vi "TLB Native Dynamic Events ver 0.14.vi"() -> ()   [LabVIEW 2018]
uses:
  Labview Training Phase 2/Enum Controls/States for Action Engine.ctl
  TLB Type Definitions/State Type Definitions.ctl
  TLB Type Definitions/Intruction Type Definitions.ctl
  TLB Type Definitions/Encoder cluster.ctl
  TLB Type Definitions/PING CLUSTER.ctl
  <vilib>/Studica/Studica Toolkit/NavX/NavX.lvlib
  <vilib>/Studica/Studica Toolkit/Background/DIO Channel.ctl
  Underlying VI's/NavX VI/navX type def.ctl
  <vilib>/myRIO/Instrument Drivers/Utilities/Utilities.lvlib
  <vilib>/Studica/Studica Toolkit/Background/I2C Channel.ctl
  TLB Type Definitions/Vision cluster.ctl
  <vilib>/NI_Real-Time Target Support.lvlib
  TLB Type Definitions/Stepper cluster.ctl
  Experimental VI's/Archived VI's/MOTOR CONTROL NO PID Type Def.ctl
  Underlying VI's/I2C Master VI/I2C MASTER Type Def.ctl
  Underlying VI's/I2C Master VI/I2C_MASTER_WRITE_NEW Type Def.ctl
  <vilib>/userdefined/High Color/IMAQdx.ctl
  Underlying VI's/I2C Master VI/Arduino_Interfacing.ctl
  TLB Type Definitions/Yaw Cluster.ctl
  Experimental VI's/Archived VI's/MOTOR CONTROL NO PID AE DATA ENTRY MODE Type def.ctl
  Experimental VI's/Archived VI's/MOTOR CONTROL NO PID AE DIRECTIONS type def.ctl
  Underlying VI's/Elasped Timer/Control.ctl
  TLB Type Definitions/Time cluster.ctl
  TLB Type Definitions/Y Stepper cluster.ctl
  Underlying VI's/Modified webcam FGV/Webcam AE.ctl
  <vilib>/Utility/RT CPU Load.ctl
panel:
  out "Object Center Coordinates":cluster{"x":sgl, "y":sgl}
  out "Object detection cluster":T1
  out "Time up flag":bool
  out "Speed & distance":T2
  out "Task selection":u8
  in  "Object recognition mode":enum16{"Ball", "Soap", "Gel", "Pipe", "None"}(ring)
  out "NavX Readings":T3
  out "Arduino Data":T4
  out "CPU loads":T5[](array[typedef]) {"ISR (%)" format="%#.2f"; "Idle (%)" format="%#.2f"; "Background (%)" format="%#.2f"; "Normal (%)" format="%#.2f"; "Above Normal (%)" format="%#.2f"; "High (%)" format="%#.2g"; "Timed Structures (%)" format="%#.2g"; "Time Critical (%)" format="%#.2g"; "Total (%)" format="%#.2g"}
  in  "Red LED":bool
  out "Obstacle detected?":bool
  out "TASK ENABLE":bool
  out "Rising Edge":bool
  in  "Green LED":bool
  out "Obstacle detected":bool
  out "I2C Error":errorcluster
  out "State Logic":T6=enum."Startup"
  out "elements":T7[](array[typedef])
  in  "STOP TASK":bool
  in  "OK Button":bool
  in  "STOP":bool
  out "error out":errorcluster
  out "Action Queue Items":i32
  out "State Logic Queue Items":i32
  out "Action Queues items":string[](array[string])=["Hardware reset", "Software reset", ""]
  out "Action State":string
  # "VISION"
  # "System Health Status Update"
  # "TLB FRAMEWORK STATUS"
  # "Test Programme written by Calvin Loke    Dated: 28 Aug 2019\nTest Programme revised by Dr Alex See   Dated 30 Aug 2019\n\nRevision date: 20/03/2020\nProgramme version:   TLB Native Dynamic Events ver 0.14"
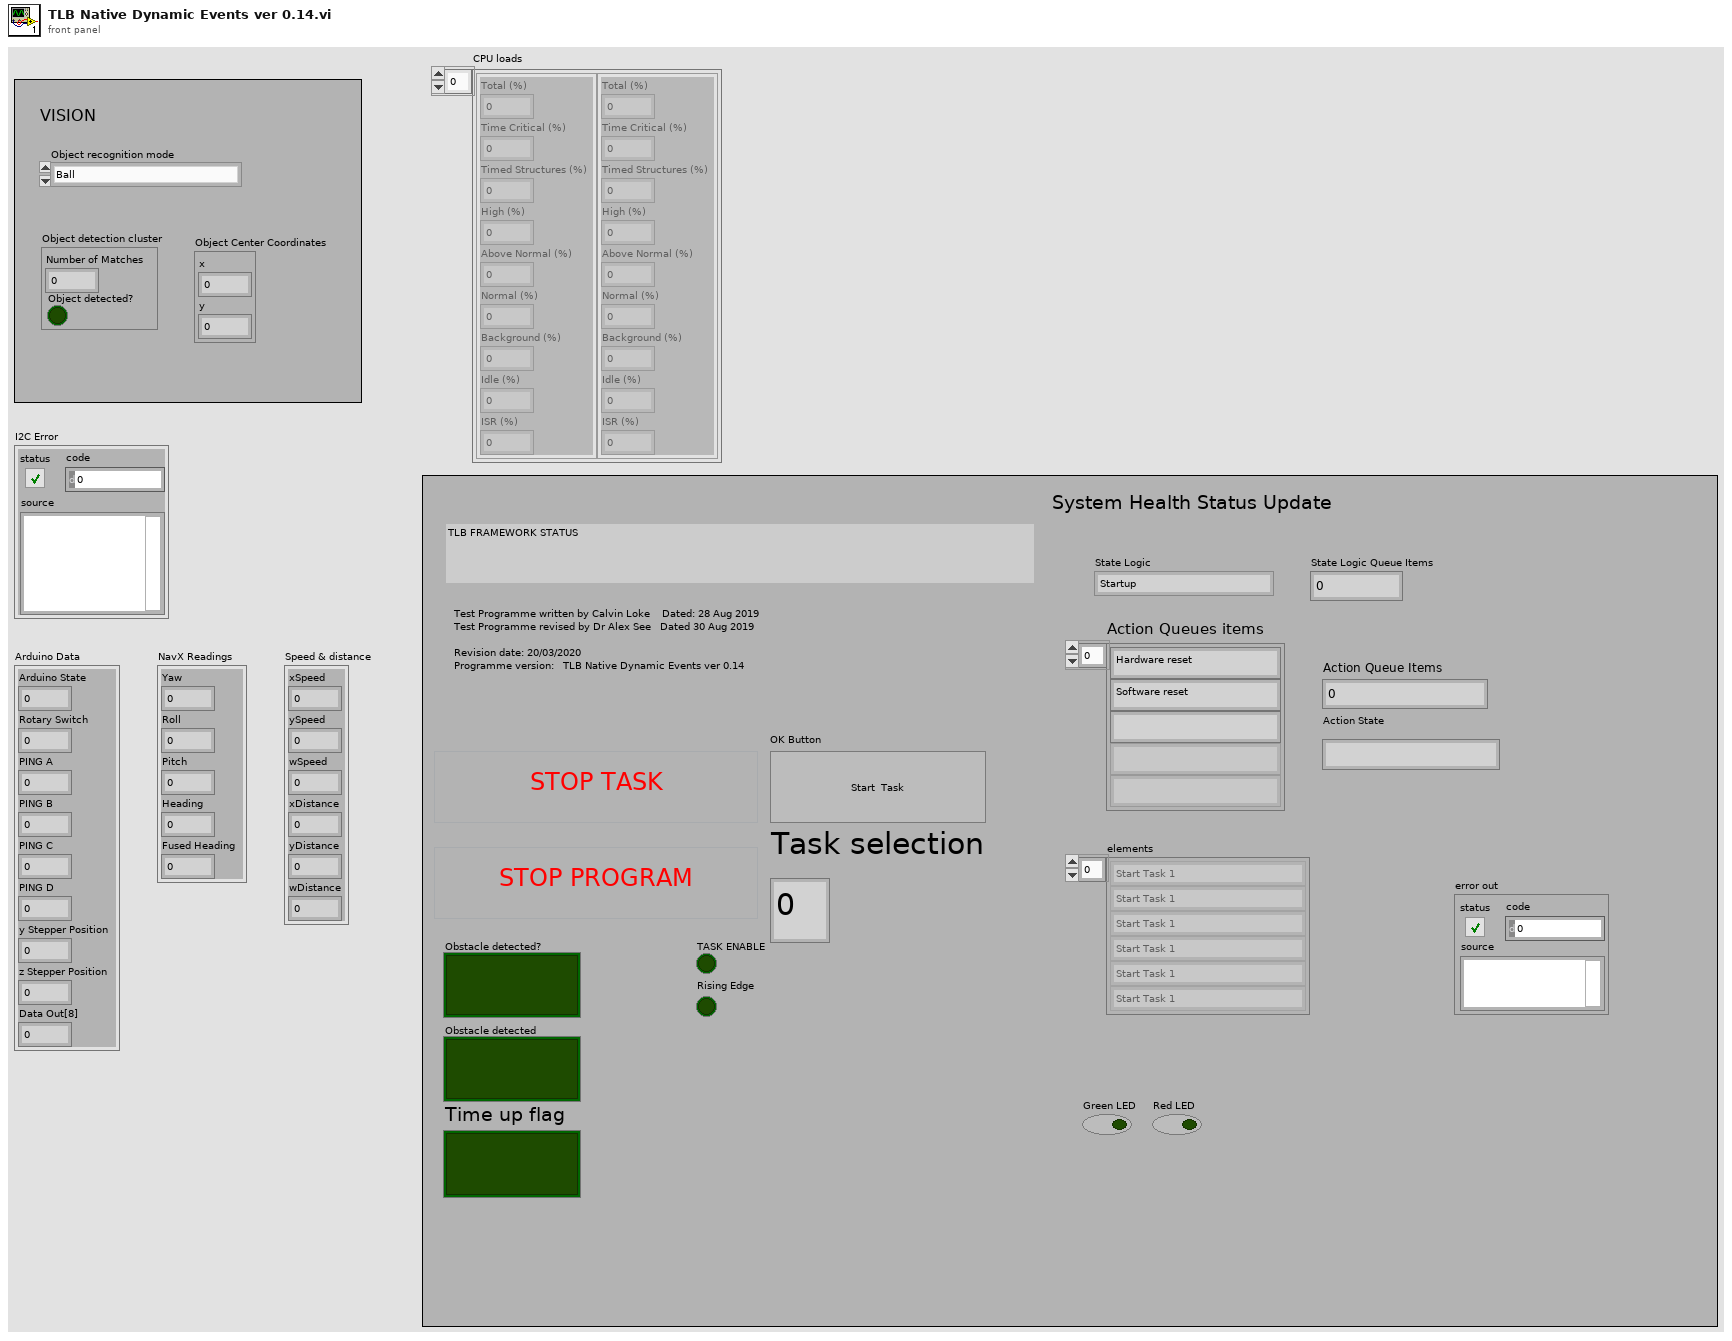
[diagram p1: front panel]
types:
  T1 = cluster{"Number of Matches":i32, "Object detected?":bool}
  T2 = cluster{"xSpeed":dbl, "ySpeed":dbl, "wSpeed":dbl, "xDistance":dbl, "yDistance":dbl, "wDistance":dbl}
  T3 = cluster{"Yaw":dbl, "Roll":dbl, "Pitch":dbl, "Heading":dbl, "Fused Heading":dbl}
  T4 = cluster{"Arduino State":u8, "Rotary Switch":u8, "PING A":u8, "PING B":u8, "PING C":u8, "PING D":u8, "y Stepper Position":u8, "z Stepper Position":u8, "Data Out[8]":u8}
  T5 = typedef "NI_Real-Time Target Support.lvlib/RT CPU Load.ctl" = cluster{"Total (%)":dbl, "Time Critical (%)":dbl, "Timed Structures (%)":dbl, "High (%)":dbl, "Above Normal (%)":dbl, "Normal (%)":dbl, "Background (%)":dbl, "Idle (%)":dbl, "ISR (%)":dbl}
  T6 = typedef "State Type Definitions.ctl" = enum16{"None", "Startup", "Move to Angle", "True Stop", "Idle", "Shutdown", "Task 1A", "Task 1B", "Task 2:Raise Arm", "Task 2:Sensor Mode", "Task 2:Reverse Mode", "Task 3", "Task 4_A", "Task 4_B", "Task 4_C", "Task 4_D", "Task 5A", "Task 5B", "Task 5C", "Task 5D", "Task 5E: POSITION ARM", "Task 5F: ARM GRAB HEIGHT", "Task 5G: CLOSE CLAW", "Task 5H: RAISE ARM", "Task 6_A", "Task 6_B", "Task 7", "Task 8A: RAISE ARM", "Task 8B: MOVE TO BOX", "Task 8C: CAM BURST", "Task 8D: PROCESS IMAGE", "Task 8E: ROBOT ADJUST", "Task 8F: CAM BURST 2", "Task 8G: PROCESS IMAGE 2", "Task 8H: ARM ADJUST", "Task 8I: ARM GRAB HEIGHT", "Task 8J: CLOSE CLAW", "Task 8K: RAISE MY SWORD", "Task 9A: Raise Arm", "Task 9B: Rotate to Angle", "Task 9C: Detect Box", "Task 9D: MOVE FORWARD", "Task 9E: MOVE LEFT", "Task 9F: SCAN IMAGE", "Task 9G: PROCESS COLOUR", "Task 9H: MOVE RIGHT", "Task 9I: SCAN IMAGE", "Task 9J: PROCESS COLOUR", "Task 9K: ROTATE 90 CW", "Task 9L: MOVE FORWARD", "Task 9M: MOVE RIGHT", "Task 9N: SCAN IMAGE", "Task 9O: PROCESS COLOUR", "Task 9P: MOVE RIGHT", "Task 9Q: SCAN IMAGE", "Task 9R: PROCESS COLOUR", "Task A1: Raise Arm", "Task A2: Rotate to Angle", "Task A3: Move Forward", "Task A4: Rotate CW 90"}
  T7 = typedef "Intruction Type Definitions.ctl" = enum16{"None", "Start Task 1", "Start Task 2", "Start Task 3", "Start Task 4", "Start Task 5", "Start Task 6", "Start Task 7", "Start Task 8 - BALL", "Start Task 8 - Gel", "Start Task 8 - Pipe", "Start Task 8 - Soap", "Start Task 9", "Start Task A", "Start Task B", "Exit"}
  T8 = typedef "Y Stepper cluster.ctl" = cluster{"yStepper desired":u8}
  T9 = typedef "Time cluster.ctl" = cluster{"Time up flag":bool, "SET TIME TO CHECK":dbl}
  T10 = typedef "Yaw Cluster.ctl" = cluster{"Yaw":dbl, "Compass":dbl}
  T11 = typedef "Stepper cluster.ctl" = cluster{"y Stepper Position":u8, "z Stepper Position":u8}
  T12 = typedef "DIO Channel.ctl" = enum16{"Not Connected", "A/DIO1", "A/DIO2", "A/DIO3", "A/DIO4", "A/DIO5", "A/DIO6", "A/DIO7", "A/DIO13", "B/DIO1", "B/DIO2", "B/DIO3", "B/DIO4", "B/DIO5", "B/DIO6", "B/DIO7", "B/DIO13", "C/DIO0", "C/DIO1", "C/DIO2", "C/DIO3", "C/DIO4", "C/DIO5", "C/DIO6", "C/DIO7"}
  T13 = typedef "Vision cluster.ctl" = cluster{"Recognized Object":bool, "Object X coordinate":dbl, "Object Y coordinate":dbl}
  T14 = typedef "PING CLUSTER.ctl" = cluster{"PING_A":u8, "PING_B":u8, "PING_C":u8, "PING_D":u8}
  T15 = typedef "Encoder cluster.ctl" = cluster{"xDistance":dbl, "yDistance":dbl, "wDistance":dbl}
  T16 = cluster{"DIO Channel":T12, "FPGA VI Reference Out":refnum<k20>}
  T17 = typedef "MOTOR CONTROL NO PID AE DATA ENTRY MODE Type def.ctl" = enum16{"Initialize", "Reset Encoders", "Write to motors", "Read from Encoders"}
  T18 = typedef "navX type def.ctl" = enum16{"Get i2C reference", "Read Values", "Zero Yaw"}
  T19 = typedef "Arduino_Interfacing.ctl" = enum16{"Initialize", "Write to Arduino", "Read From Arduino"}
  T20 = typedef "I2C Channel.ctl" = enum16{"Not Connected", "A", "B"}
  T21 = typedef "States for Action Engine.ctl" = enum16{"Initialize", "Write", "Read"}
  T22 = cluster{"I2C Ref Out":cluster{"I2C Channel":T20, "FPGA VI Reference Out":refnum<k20>}, "Connected":bool, "Slave Address (7-bit)":u8, "Registry":u8[]}
  T23 = typedef "IMAQ Image.ctl" = refnum<image>
  T24 = typedef "State Type Definitions.ctl" = enum16{"None", "Startup", "Move to Angle", "True Stop", "Idle", "Shutdown", "Task 1", "Task 2", "Task 3", "Task 4_A", "Task 4_B", "Task 4_C", "Task 4_D", "Task 5_A", "Task 5 _B", "Task 5_C", "Task 5_D", "Task 5_D_Error", "Task 5D_Error_Right", "Task 5D_Error_Left", "Task 5_E", "Task 5_F", "Task 5F_Error", "Task 5G", "Task 5H", "Task 6_A", "Task 6_B", "Task 7", "Task 8", "Task 9", "Task A", "Task B"}
  T25 = typedef "State Type Definitions.ctl" = enum16{"None", "Startup", "Move to Angle", "True Stop", "Idle", "Shutdown", "Task 1", "Task 2", "Task 3", "Task 4_A", "Task 4_B", "Task 4_C", "Task 5_A", "Task 5 _B", "Task 5_C", "Task 5_C_Error", "Task 6_A", "Task 6_B", "Task 7", "Task 8", "Task 9", "Task A", "Task B"}
  T26 = typedef "MOTOR CONTROL NO PID AE DIRECTIONS type def.ctl" = enum16{"y-axis movement", "x-axis movement", "Rotate", "Stop"}
  T27 = typedef "Control.ctl" = enum16{"Start", "Pause", "Initialize"}
  T28 = typedef "I2C_MASTER_WRITE_NEW Type Def.ctl" = enum16{"Ultrasonic sensors", "Stepper origin", "zStepper 13.3k", "zStepper 13k", "zStepper 12k", "zStepper 11k", "zStepper 10k", "zStepper 9k", "zStepper 8k", "zStepper 7k", "zStepper 6k", "zStepper 5k", "zStepper 4k", "zStepper 3k", "zStepper 2k", "zStepper 1k", "zStepper 900", "zStepper 800", "zStepper 700", "zStepper 600", "zStepper 500", "zStepper 400", "zStepper 300", "zStepper 200", "zStepper 100", "zStepper 0", "yStepper control", "Open Claw", "Close Claw", "Soft Reset"}
  T29 = typedef "Webcam AE.ctl" = enum16{"Initialize Camera", "Open Camera", "Continuous Acquisition", "Close Camera", "Retrieve Image", "Dispose Camera Image Buffer"}
  T30 = typedef "IMAQdx.ctl" = refnum<k21>
  T31 = typedef "Webcam AE.ctl" = enum16{"Initialize Camera", "Open Camera", "Continuous Acquisition", "Close Camera", "Retrieve Image", "Dispose Image Buffers"}
  T32 = typedef "MOTOR CONTROL NO PID Type Def.ctl" = enum16{"Init", "Front Back", "Left Right", "Rotate", "Stop", "Latch"}
  T33 = typedef "I2C MASTER Type Def.ctl" = enum16{"Last State", "Mode 0", "Mode 1", "Mode 2", "Mode 3", "Mode 4", "Mode 5", "Mode 6", "Mode 7", "Mode 8", "Mode 9", "Mode 10"}
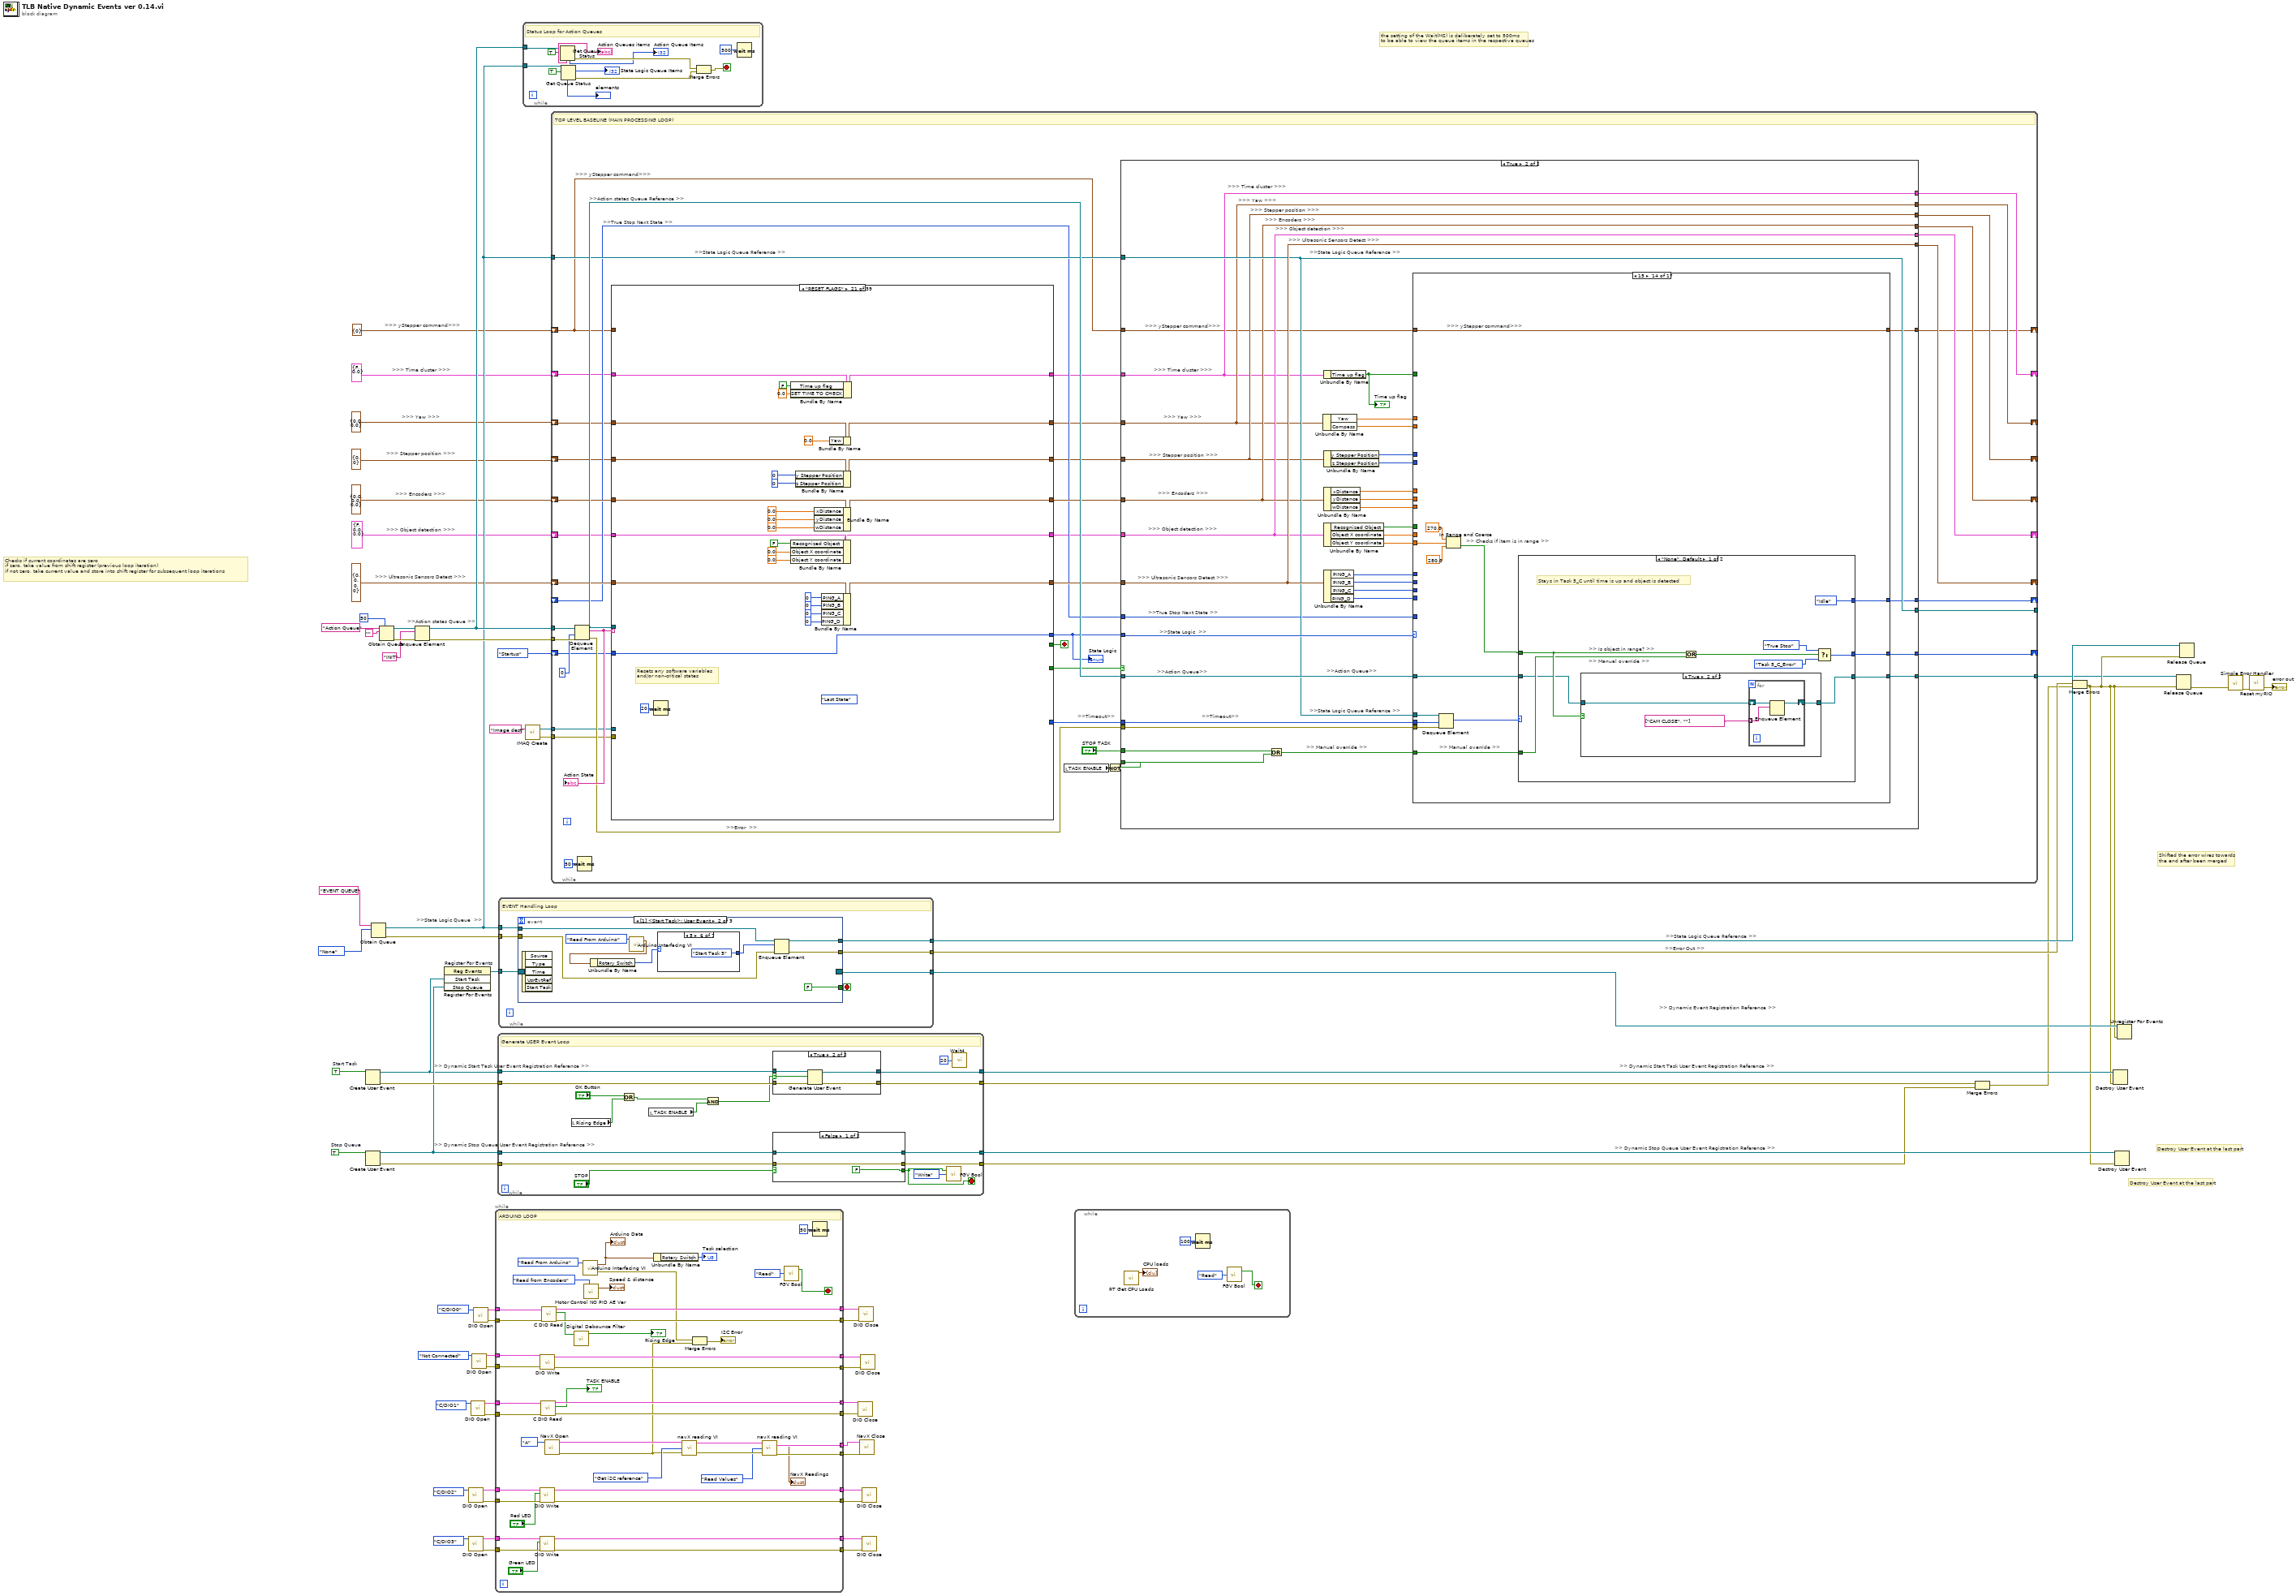
[diagram p0: block diagram]
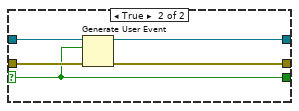
[diagram p2: hidden frame]
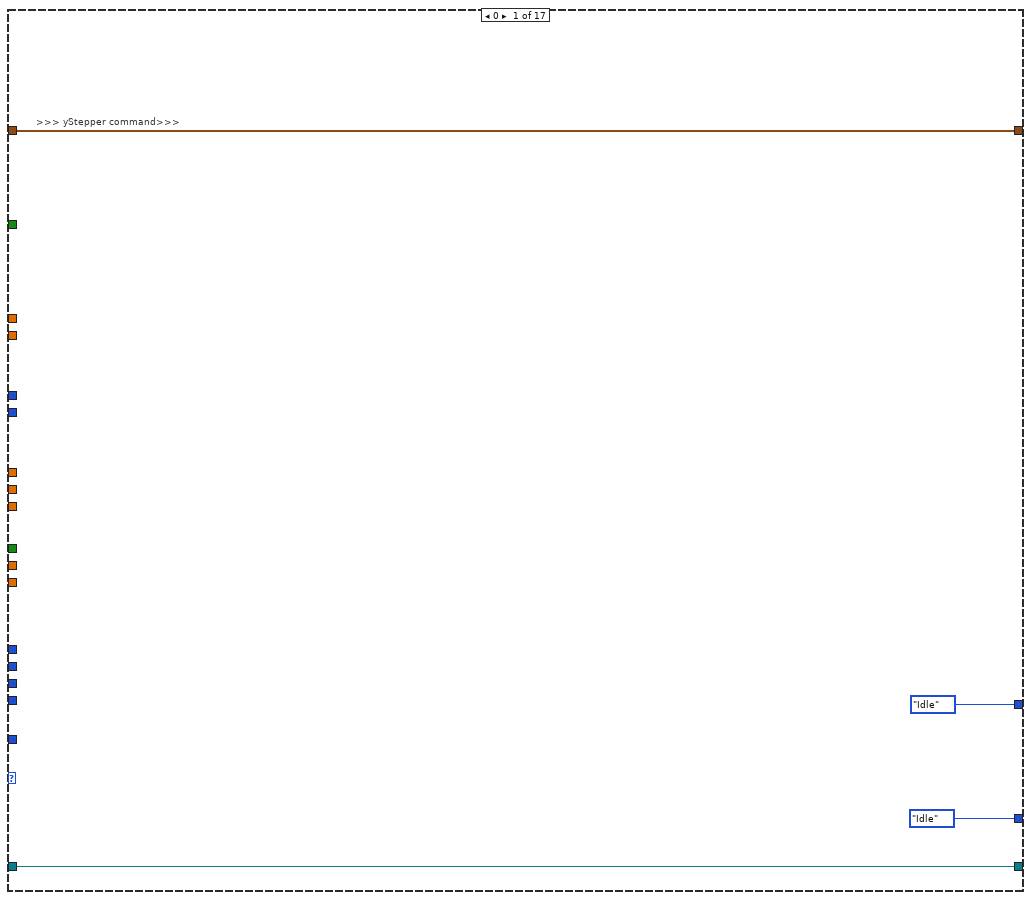
[diagram p5: hidden frame]
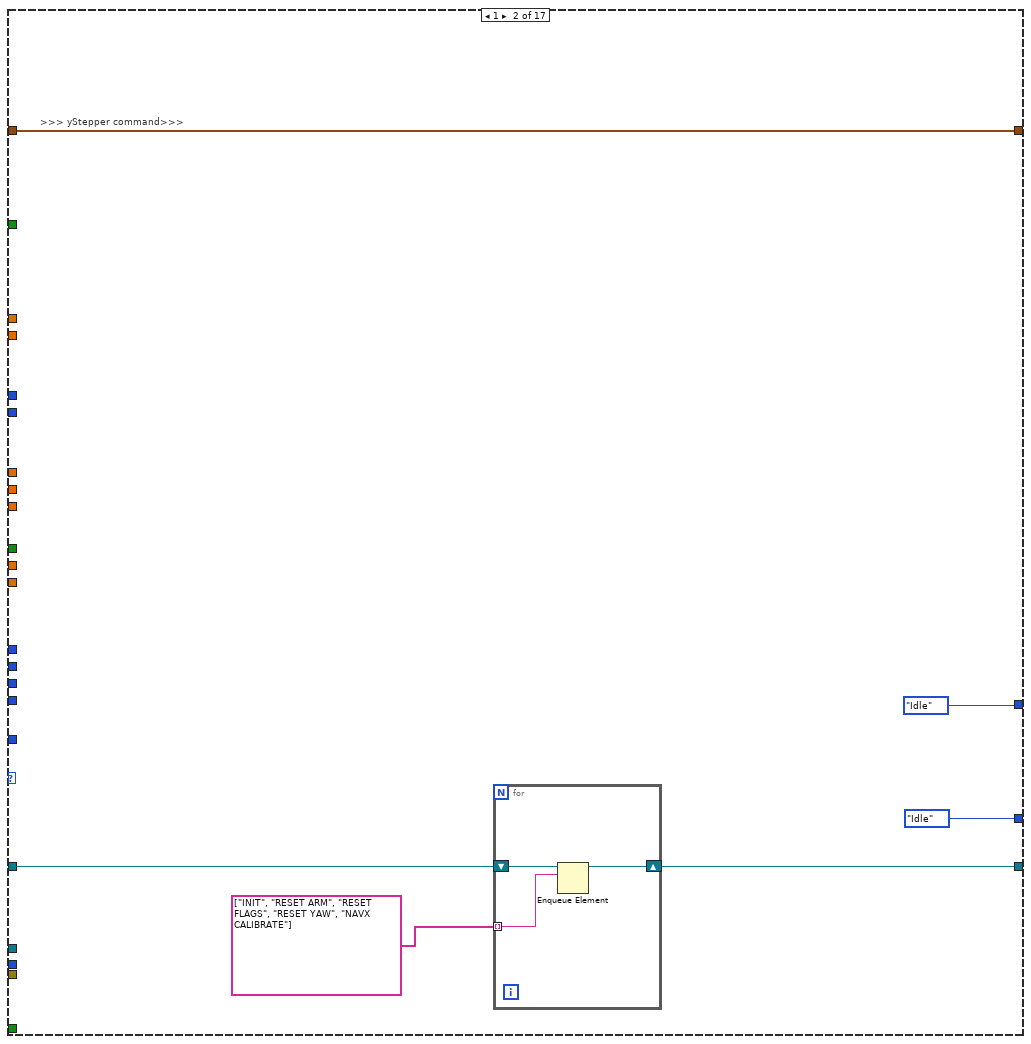
[diagram p6: hidden frame]
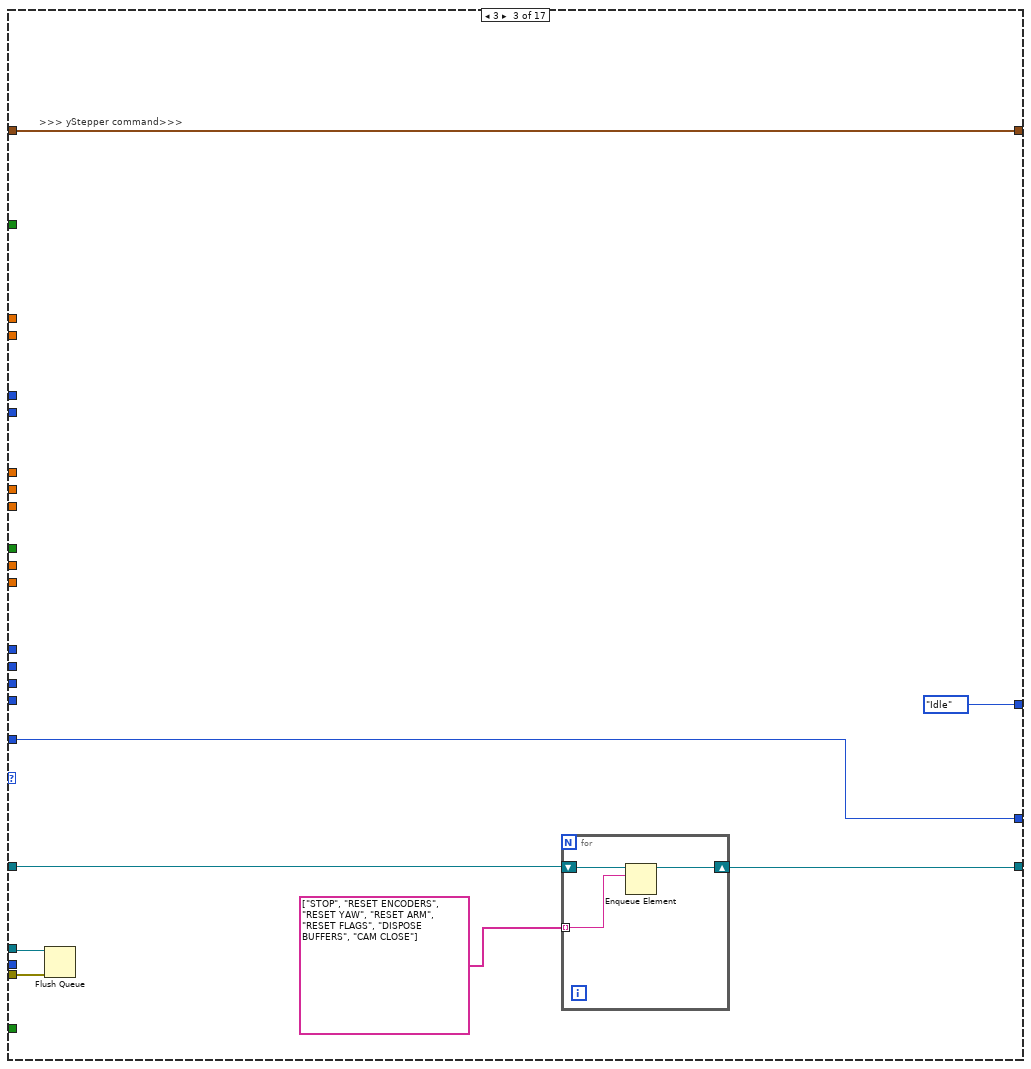
[diagram p7: hidden frame]
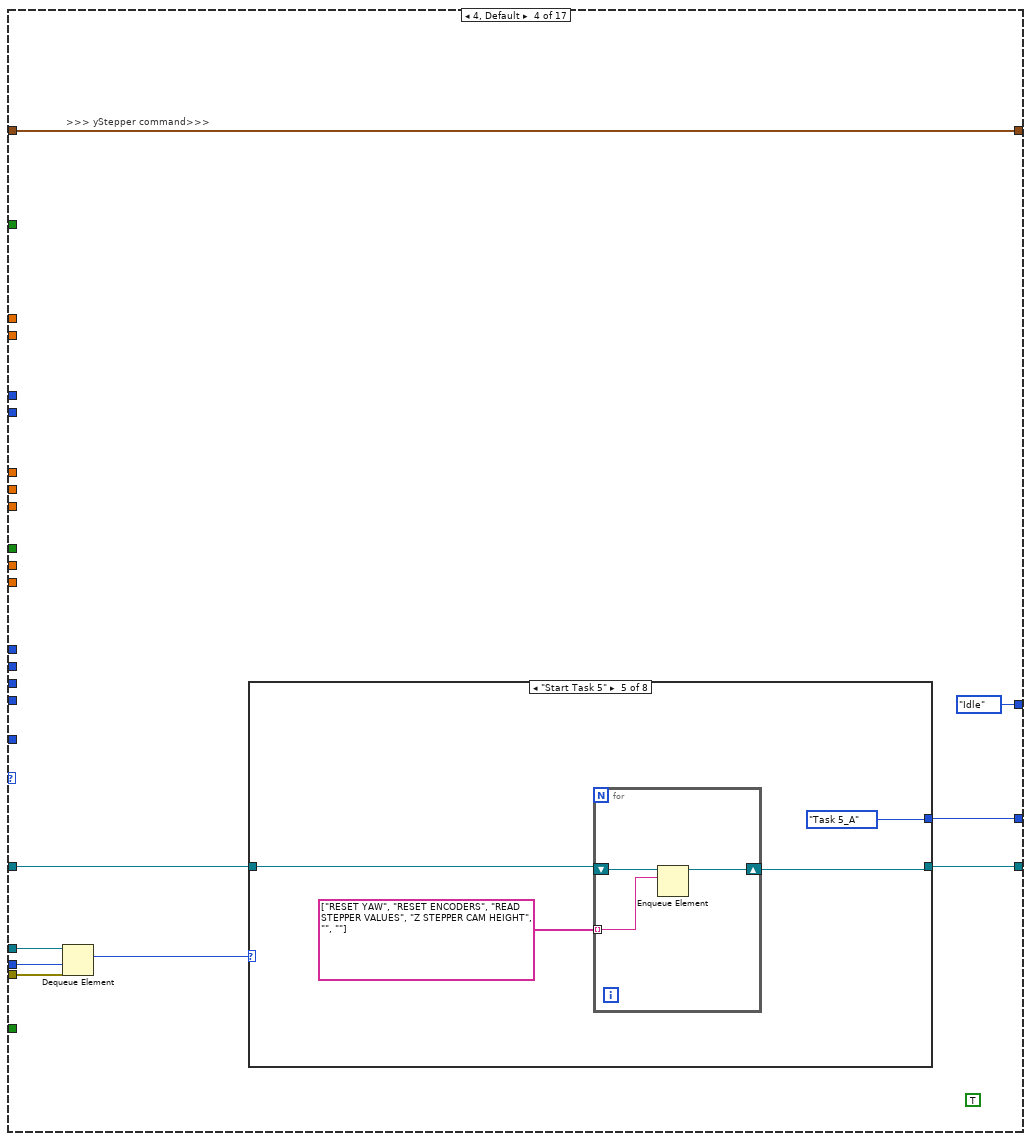
[diagram p8: hidden frame]
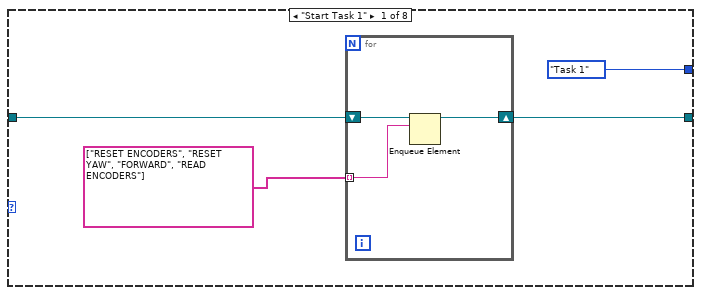
[diagram p9: hidden frame]
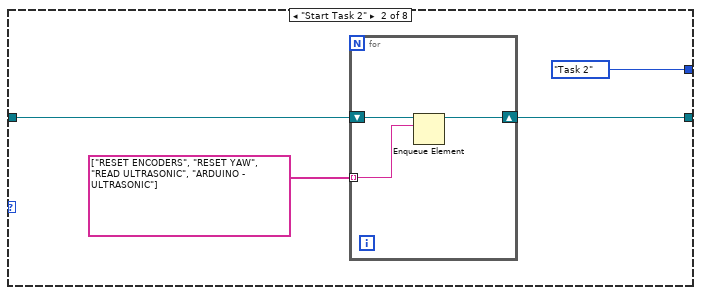
[diagram p10: hidden frame]
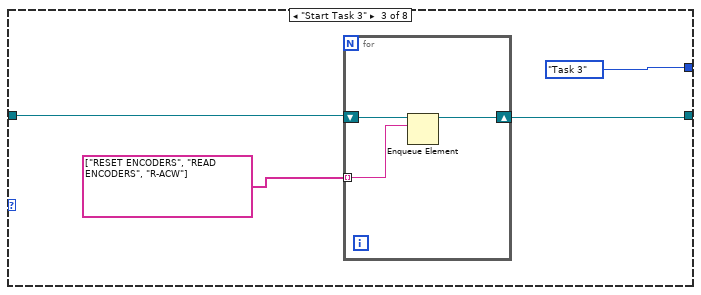
[diagram p11: hidden frame]
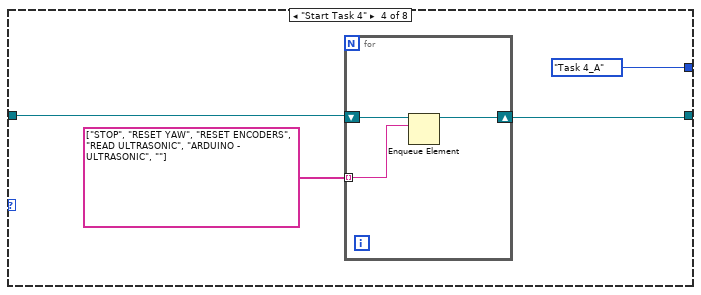
[diagram p12: hidden frame]
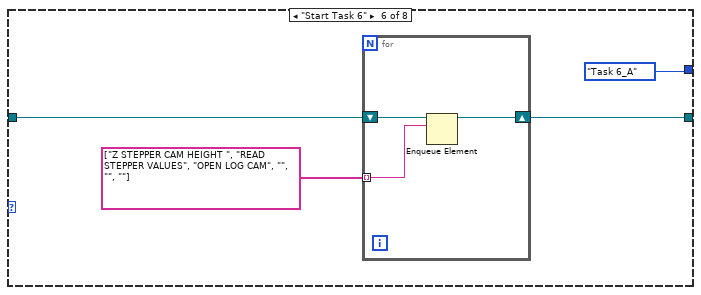
[diagram p13: hidden frame]
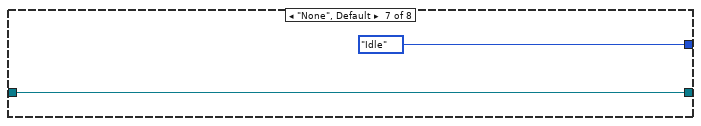
[diagram p14: hidden frame]
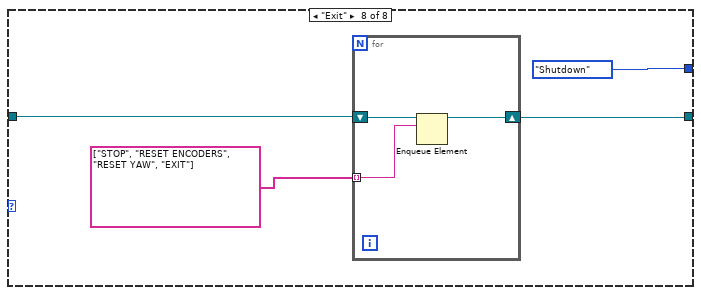
[diagram p15: hidden frame]
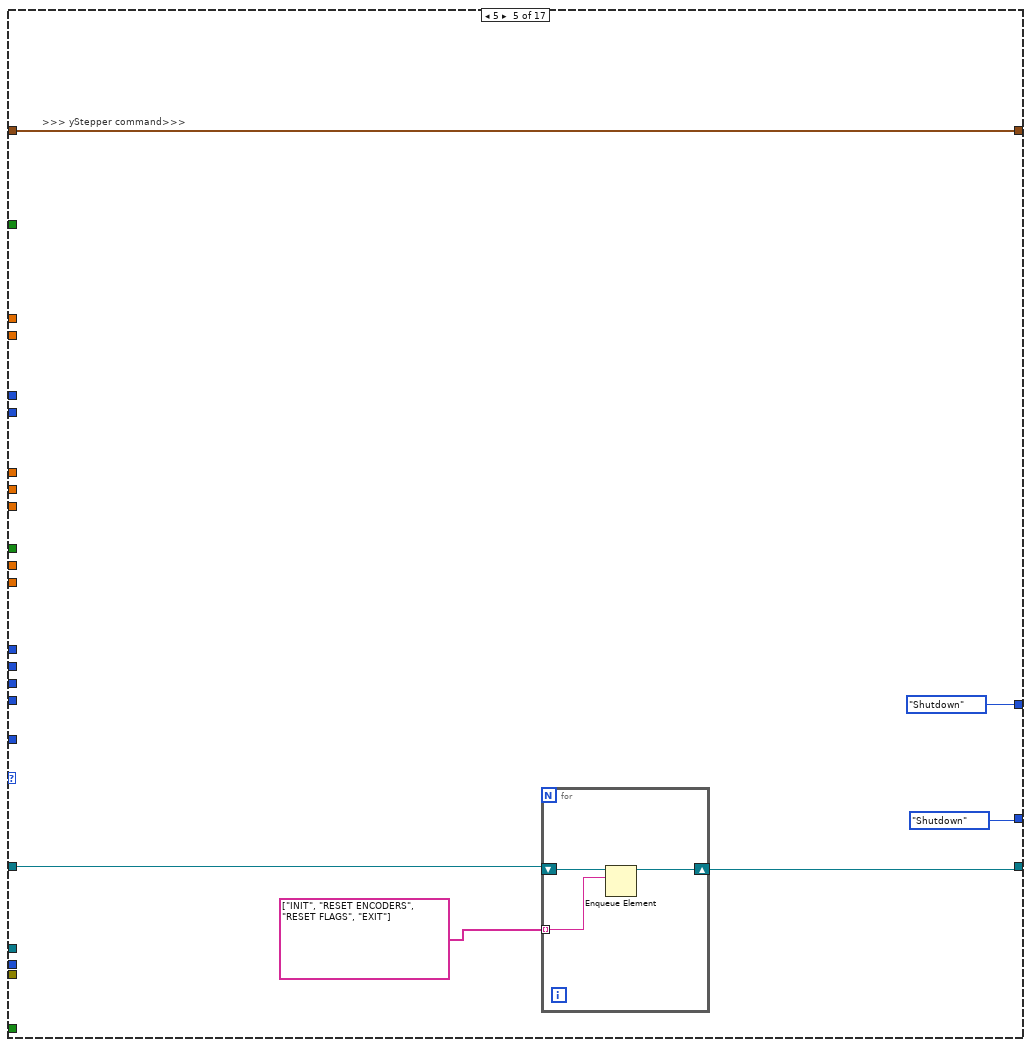
[diagram p16: hidden frame]
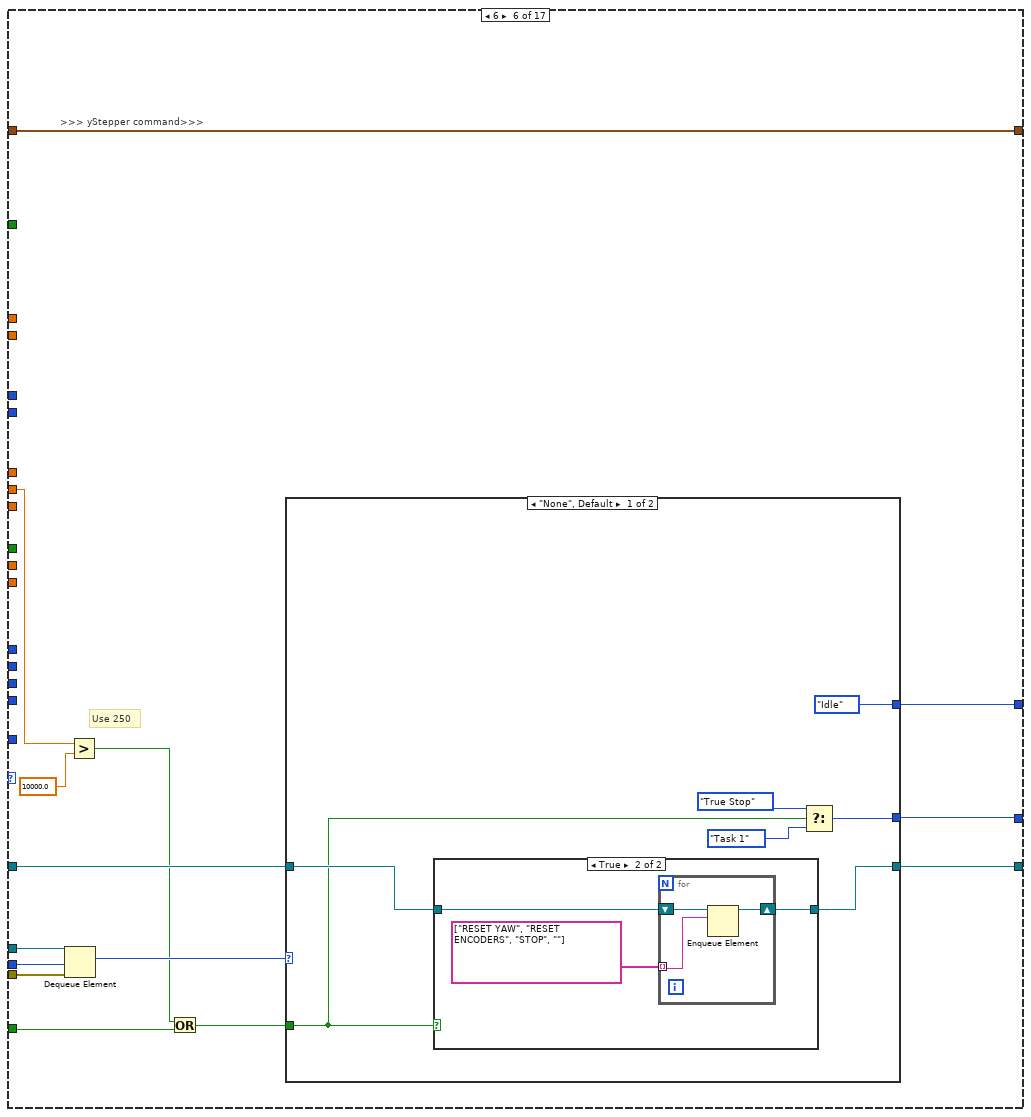
[diagram p17: hidden frame]
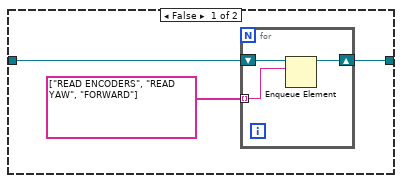
[diagram p18: hidden frame]
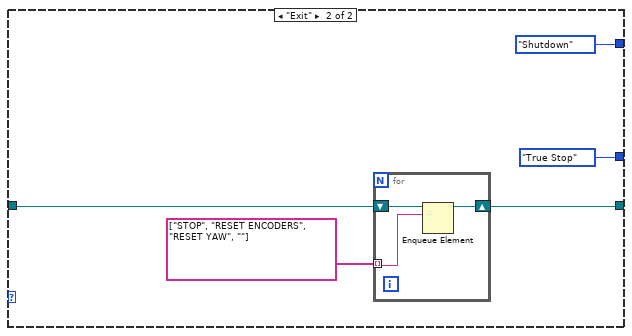
[diagram p19: hidden frame]
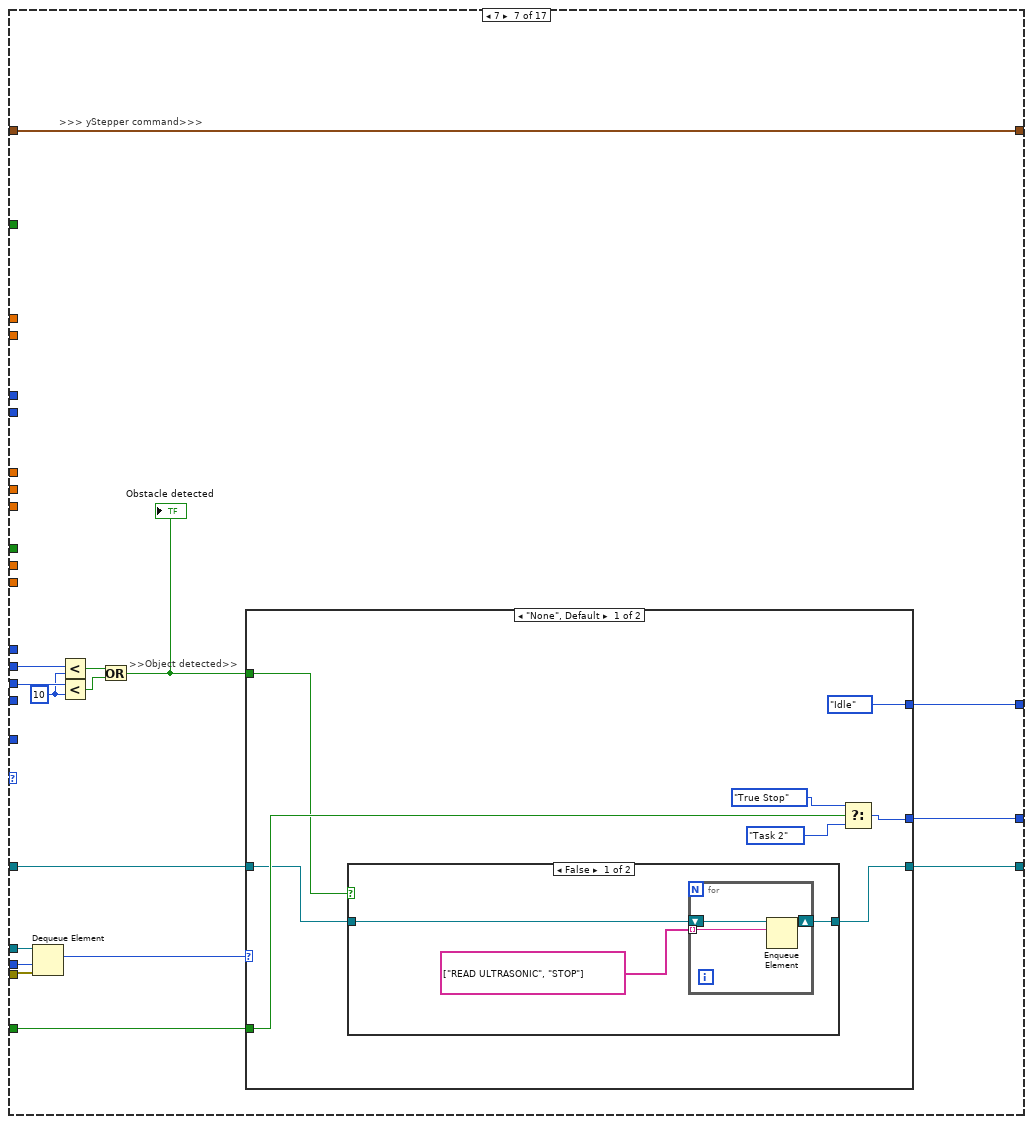
[diagram p20: hidden frame]
diagram:
  w70 = TRUE  # Stop Queue
  w69 = TRUE  # Start Task
  # "Checks if current coordinates are zero\nif zero, take value from shift register (previous loop iteration)\nif not zero, take current value and store into shift register for subsequent loop iterations"
  # ">>> yStepper command>>>"
  # ">>> Time cluster >>>"
  # ">>> Yaw >>>"
  # ">>> Stepper position >>>"
  # ">>> Encoders >>>"
  # ">>> Object detection >>>"
  # ">>> Ultrasonic Sensors Detect >>>"
  # "the setting of the Wait(MS) is deliberately set to 500ms\nto be able to view the queue items in the respective queues"
  # ">>Error Out >>"
  # ">> Dynamic Stop Queue User Event Registration Reference >>"
  # ">> Dynamic Start Task User Event Registration Reference >>"
  # ">> Dynamic Stop Queue User Event Registration Reference >>"
  # ">> Dynamic Start Task User Event Registration Reference >>"
  # ">> Dynamic Event Registration Reference >>"
  # ">>Action states Queue >>"
  # ">>State Logic Queue  >>"
  # ">>State Logic Queue Reference >>"
  # "Destroy User Event at the last part"
  # "Destroy User Event at the last part"
  # "Shifted the error wires towards\nthe end after been merged"
  n1 = Create User Event(user event datatype=w69) -> (user event=w61:refnum<user-event>, error out=w66:errorcluster)  [unwired: 1 in]
  n2 = Create User Event(user event datatype=w70) -> (user event=w62:refnum<user-event>, error out=w65:errorcluster)  [unwired: 1 in]
  n3 = Obtain Queue(name (unnamed)="EVENT QUEUE", element data type=Intruction_Type_Definitions."None" ("Enum")) -> (queue out=w47:refnum<queue>, error out=w53:errorcluster)  [unwired: 3 in, 1 out]
  n4 = Obtain Queue(max queue size (-1, unlimited)=50, name (unnamed)="Action Queue", element data type="") -> (queue out=w56:refnum<queue>, error out=w52:errorcluster)  [unwired: 2 in, 1 out]
  n5 = Enqueue Element(queue=w56, element="INIT", error in (no error)=w52) -> (queue out=w48:refnum<queue>, error out=w51:errorcluster)  [unwired: 1 in, 1 out]
  n6 = register-events "Register For Events"(w61, w62) -> (reference out=w60:refnum<event-registration>)  [unwired: 2 in, 1 out]
  n7 = call <vilib>:"DIO Open.vi"("DIO Channel"=DIO_Channel."C/DIO2") -> ("error out"=w14:errorcluster, "DIO Info Out"=w15:T16)  [unwired: 9 in]
  n8 = call <vilib>:"DIO Open.vi"("DIO Channel"=DIO_Channel."C/DIO3") -> ("error out"=w9:errorcluster, "DIO Info Out"=w10:T16)  [unwired: 9 in]
  n9 = call <vilib>:"DIO Open.vi"("DIO Channel"=DIO_Channel."C/DIO1") -> ("error out"=w25:errorcluster, "DIO Info Out"=w26:T16)  [unwired: 9 in]
  n10 = call <vilib>:"DIO Open.vi"("DIO Channel"=DIO_Channel."Not Connected") -> ("error out"=w30:errorcluster, "DIO Info Out"=w32:T16)  [unwired: 9 in]
  n11 = call <vilib>:"DIO Open.vi"("DIO Channel"=DIO_Channel."C/DIO0") -> ("error out"=w35:errorcluster, "DIO Info Out"=w38:T16)  [unwired: 9 in]
  n12 = while {
    tunnel: w38 -> [w112]
    tunnel: [w111] -> w36
    tunnel: w35 -> [w110]
    tunnel: [w109] -> w34
    tunnel: w32 -> [w105]
    tunnel: [w104] -> w31
    tunnel: w30 -> [w103]
    tunnel: [w102] -> w29
    tunnel: [w101] -> w27
    tunnel: w26 -> [w100]
    tunnel: w25 -> [w99]
    tunnel: [w98] -> w24
    tunnel: w15 -> [w92]
    tunnel: w14 -> [w91]
    tunnel: [w90] -> w13
    tunnel: [w89] -> w12
    tunnel: w10 -> [w87]
    tunnel: w9 -> [w86]
    tunnel: [w85] -> w8
    tunnel: [w84] -> w7
    tunnel: [w78] -> w4
    tunnel: [w77] -> w5
    stop <- w114 stop-if-true
    # "ARDUINO LOOP"
    n13 = call <vilib>:"DIO Write.vi"("error in (no error)"=w91, "Input"="Red LED", "DIO Info In"=w92) -> ("error out"=w89:errorcluster, "DIO Info Out"=w90:T16)  [unwired: 7 in]
    n14 = call <vilib>:"DIO Write.vi"("error in (no error)"=w86, "Input"="Green LED", "DIO Info In"=w87) -> ("error out"=w84:errorcluster, "DIO Info Out"=w85:T16)  [unwired: 7 in]
    n15 = call <vilib>:"DIO Write.vi"("error in (no error)"=w103, "DIO Info In"=w105) -> ("error out"=w102:errorcluster, "DIO Info Out"=w104:T16)  [unwired: 8 in]
    n16 = call <vilib>:"C DIO Read.vi"("error in (no error)"=w99, "DIO Info In in"=w100) -> ("error out"=w98:errorcluster, "IN"=→"TASK ENABLE":bool, "DIO Info In out"=w101:T16)  [unwired: 7 in]
    n17 = call <vilib>:"C DIO Read.vi"("error in (no error)"=w110, "DIO Info In in"=w112) -> ("error out"=w109:errorcluster, "IN"=w107:bool, "DIO Info In out"=w111:T16)  [unwired: 7 in]
    n18 = call <vilib>:"NavX Open.vi"("I2C Channel"=I2C_Channel."A") -> ("error out"=w94:errorcluster, "NavX Info"=w96:T22)  [unwired: 9 in]
    n19 = call "Digital Debounce Filter.vi"("Boolean input"=w107) -> ("Rising Edge"=→"Rising Edge":bool)  [unwired: 1 in, 2 out]
    n20 = call "Arduino Interfacing VI.vi"("AE Mode"=Arduino_Interfacing."Read From Arduino") -> ("error out"=w81:errorcluster, "Arduino Data"=w74:T4)  [unwired: 3 in]
    "Arduino Data" <- w74
    n21 = call "Motor Control NO PID AE Ver.vi"("AE Mode"=MOTOR_CONTROL_NO_PID_AE_DATA_ENTRY_MODE_Type_def."Read from Encoders") -> ("Speed & distance"=→"Speed & distance":T2)  [unwired: 4 in, 1 out]
    n22 = Unbundle By Name(w74) -> ("Rotary Switch"=→"Task selection":u8)
    n23 = call "navX reading VI.vi"("NavX Info In"=w96, "Mode"=navX_type_def."Get i2C reference", "error in (no error)"=w94) -> ("NavX Info Out"=w80:T22, "Error Out"=w79:errorcluster)  [unwired: 2 out]
    n24 = Merge Errors(w81, w94) -> (→"I2C Error":errorcluster)
    n25 = call "navX reading VI.vi"("NavX Info In"=w80, "Mode"=navX_type_def."Read Values", "error in (no error)"=w79) -> ("NavX Info Out"=w78:T22, "NavX Readings"=→"NavX Readings":T3, "Error Out"=w77:errorcluster)  [unwired: 1 out]
    n26 = call "FGV Bool.vi"("Init/Read/Write State"=States_for_Action_Engine."Read") -> ("Output node"=w114:bool)  [unwired: 2 in, 1 out]
    n27 = Wait (ms)(milliseconds to wait=u32 50) -> ()  [unwired: 1 out]
  }
  n28 = while {
    tunnel: w61 -> [w132]
    tunnel: w62 -> [w131]
    tunnel: [w130] -> w68
    tunnel: [w129] -> w67
    tunnel: w66 -> [w128]
    tunnel: [w127] -> w64
    tunnel: w65 -> [w126]
    tunnel: [w125] -> w63
    stop <- w123 stop-if-true
    # "Generate USER Event Loop"
    n29 = local read "Rising Edge"() -> (w119:bool)
    n30 = Or(x="OK Button", y=w119) -> (x .or. y?=w118:bool)
    n31 = local read "TASK ENABLE"() -> (w117:bool)
    n32 = And(x=w118, y=w117) -> (x .and. y?=w116:bool)
    n33 = case shown="True" w116 {
      selector: w116 -> [_ w143]
      tunnel: w132 -> [w142 w147]
      tunnel: [w142 w146] -> w129
      tunnel: w128 -> [w141 w145]
      tunnel: [w141 w144] -> w127
      frame False {
      }
      frame True {
        n34 = Generate User Event(user event=w147, event data cluster=w143, error in=w145) -> (user event out=w146:refnum<user-event>, error out=w144:errorcluster)  [unwired: 1 in]
      }
    }
    n35 = case shown="False" "STOP" {
      selector: "STOP" -> [_ w136]
      tunnel: w131 -> [w135 w140]
      tunnel: [w135 w139] -> w130
      tunnel: w126 -> [w134 w138]
      tunnel: [w134 w137] -> w125
      tunnel: [FALSE w136] -> w123
      frame False {
      }
      frame True {
        n36 = Generate User Event(user event=w140, event data cluster=w136, error in=w138) -> (user event out=w139:refnum<user-event>, error out=w137:errorcluster)  [unwired: 1 in]
      }
    }
    n37 = call "FGV Bool.vi"("Init/Read/Write State"=States_for_Action_Engine."Write", "Input Node"=w123) -> ()  [unwired: 1 in, 2 out]
    n38 = call "Wait4"("Count(uSec)"=u32 20) -> ()  [unwired: 1 out]
  }
  n39 = while {
    tunnel: w60 -> [w154]
    tunnel: [w153] -> w59
    tunnel: w47 -> [w151]
    tunnel: [w150] -> w58
    tunnel: w53 -> [w149]
    tunnel: [w148] -> w50
    stop <- w152 stop-if-true
    # "EVENT Handling Loop"
    n40 = event shown="[1] <Start Task>: User Event" {
      selector: w154 -> [_ _ _]
      dyn-events: [_ _ _] -> w153
      timeout: _ -> [_ _ _]
      tunnel: [FALSE FALSE w182] -> w152
      tunnel: w151 -> [w159 w168 w180]
      tunnel: [w158 w167 w181] -> w150
      tunnel: w149 -> [w157 w166 w179]
      tunnel: [w156 w165 w178] -> w148
      event Timeout {
        n41 = event-data() -> ()  [unwired: 1 in, 3 out]
        n42 = Enqueue Element(queue=w159, element=Intruction_Type_Definitions."None" ("Enum"), error in (no error)=w157) -> (queue out=w158:refnum<queue>, error out=w156:errorcluster)  [unwired: 1 in, 1 out]
      }
      event User Event {
        n43 = event-data() -> ()  [unwired: 1 in, 5 out]
        n44 = call "Arduino Interfacing VI.vi"("AE Mode"=Arduino_Interfacing."Read From Arduino") -> ("Arduino Data"=w162:T4)  [unwired: 3 in, 1 out]
        n45 = Unbundle By Name(w162) -> ("Rotary Switch"=w161:u8)
        n46 = case shown="5" w161 {
          tunnel: [Intruction_Type_Definitions."None" ("Enum") Intruction_Type_Definitions."Start Task 1" ("Enum") Intruction_Type_Definitions."Start Task 2" ("Enum") Intruction_Type_Definitions."Start Task 3" ("Enum") Intruction_Type_Definitions."Start Task 4" ("Enum") Intruction_Type_Definitions."Start Task 5" ("Enum") Intruction_Type_Definitions."Start Task 6" ("Enum")] -> w164
          frame 0, Default {
          }
          frame 1 {
          }
          frame 2 {
          }
          frame 3 {
          }
          frame 4 {
          }
          frame 5 {
          }
          frame 6 {
          }
        }
        n47 = Enqueue Element(queue=w168, element=w164, error in (no error)=w166) -> (queue out=w167:refnum<queue>, error out=w165:errorcluster)  [unwired: 1 in, 1 out]
      }
      event User Event {
        n48 = event-data() -> ("Stop Queue"=w182:bool)  [unwired: 1 in, 4 out]
        n49 = Enqueue Element At Opposite End(queue=w180, element=Intruction_Type_Definitions."Exit" ("Enum"), error in (no error)=w179) -> (queue out=w181:refnum<queue>, error out=w178:errorcluster)  [unwired: 1 in, 1 out]
      }
    }
  }
  n50 = while {
    tunnel: w48 -> [w192]
    tunnel: w47 -> [w189]
    stop <- w186 stop-if-true
    # "Status Loop for Action Queues"
    n51 = Get Queue Status(queue=w192, return elements? (F)=TRUE) -> (error out=w188:errorcluster, # elements in queue=→"Action Queue Items":i32, elements=→"Action Queues items":string[])  [unwired: 1 in, 5 out]
    n52 = Get Queue Status(queue=w189, return elements? (F)=TRUE) -> (# pending remove=→"State Logic Queue Items":i32, error out=w187:errorcluster, elements=→"elements":T7[])  [unwired: 1 in, 5 out]
    n53 = Merge Errors(w188, w187) -> (w186:errorcluster)
    n54 = Wait (ms)(milliseconds to wait=u32 500) -> ()  [unwired: 1 out]
  }
  n55 = call "IMAQ Create"("Image Name"="Image dest") -> ("New Image"=w19:T23, "error out"=w18:errorcluster)  [unwired: 4 in]
  n56 = while {
    tunnel: w47 -> [w225]
    tunnel: w48 -> [w237]
    tunnel: w51 -> [w235]
    tunnel: [w234] -> _
    tunnel: [w233] -> w41
    shift-right: [w226] -> _
    shift-left: T14 {"PING_A"=0, "PING_B"=0, "PING_C"=0, "PING_D"=0} -> [w228]
    shift-right: [w219] -> _
    shift-left: State_Type_Definitions."Startup" ("Enum") -> [w222]
    shift-right: [w215] -> _
    shift-left: T15 {"xDistance"=0.0, "yDistance"=0.0, "wDistance"=0.0} -> [w217]
    shift-right: [w212] -> _
    shift-left: _ -> [w211]
    tunnel: w19 -> [w210]
    tunnel: w18 -> [w209]
    shift-right: [w206] -> _
    shift-left: T13 {"Recognized Object"=FALSE, "Object X coordinate"=0.0, "Object Y coordinate"=0.0} -> [w208]
    shift-right: [w203] -> _
    shift-left: T11 {"y Stepper Position"=0, "z Stepper Position"=0} -> [w205]
    shift-right: [w200] -> _
    shift-left: T10 {"Yaw"=0.0, "Compass"=0.0} -> [w202]
    shift-right: [w197] -> _
    shift-left: T9 {"Time up flag"=FALSE, "SET TIME TO CHECK"=0.0} -> [w199]
    shift-right: [w195] -> _
    shift-left: T8 {"yStepper desired"=0} -> [w196]
    stop <- w224 stop-if-true
    # ">>> yStepper command>>>"
    # ">>True Stop Next State >>"
    # ">>Error  >>"
    # ">>Timeout>>"
    # ">>Action states Queue Reference >>"
    # ">>State Logic Queue Reference >>"
    # "TOP LEVEL BASELINE (MAIN PROCESSING LOOP)"
    n57 = Dequeue Element(queue=w237, timeout in ms (-1)=0, error in (no error)=w235) -> (queue out=w229:refnum<queue>, element=w236:string, error out=w230:errorcluster)  [unwired: 1 out]
    "Action State" <- w236
    n58 = Wait (ms)(milliseconds to wait=u32 50) -> ()  [unwired: 1 out]
    n59 = case shown="\"RESET FLAGS\"" w236 {
      tunnel: [_ _ _ _ _ _ _ _ _ _ _ _ _ _ _ _ 0 w1102 _ _ _ _ _ _ _ _ _ _ _ _ _ _ _ _ _ _ _ _ _] -> w232
      tunnel: w229 -> [_ _ _ _ _ _ _ _ _ _ _ _ _ _ _ _ _ _ _ _ _ _ _ _ _ _ _ _ _ _ _ _ _ _ _ _ _ _ _]
      tunnel: w228 -> [w917 w925 w936 w947 w957 w967 w978 w989 w999 w1005 w1019 w1032 w1043 w1051 w1075 w1084 w1094 w1103 w1111 w1119 w1148 w1158 w1165 w1173 w1185 w1197 w1206 w1214 w1230 w1238 w1248 w1257 w1266 w1275 w1283 w1298 w1303 w1314 w1324]
      tunnel: [w917 w925 w936 w947 w957 w967 w978 w989 w999 w1005 w1019 w1033 w1043 w1051 w1076 w1084 w1094 w1103 w1111 w1119 w1147 w1158 w1165 w1173 w1185 w1197 w1206 w1214 w1230 w1238 w1248 w1257 w1266 w1275 w1283 w1298 w1303 w1314 w1324] -> w227
      tunnel: [TRUE TRUE _ _ _ _ _ _ _ _ _ _ _ _ _ _ _ _ _ _ _ _ _ _ _ _ _ _ _ _ _ _ _ _ _ _ _ _ _] -> w224
      tunnel: w222 -> [w915 w923 w935 w946 w956 w966 w977 w988 w998 w1004 w1018 w1031 w1042 w1050 w1074 w1083 w1091 w1100 w1110 w1118 w1146 w1157 w1164 w1172 w1184 w1196 w1205 w1213 w1229 w1237 w1247 w1256 w1265 w1274 w1282 w1297 w1302 w1313 w1323]
      tunnel: [_ _ _ _ _ _ _ _ _ _ _ _ _ _ _ _ _ TRUE _ _ _ _ _ _ _ _ _ _ _ _ _ _ _ _ _ _ _ _ _] -> w221
      tunnel: [w915 w923 w935 w946 w956 w966 w977 w988 w998 w1004 w1018 w1031 w1042 w1050 w1074 w1083 w1091 w1100 w1110 w1118 w1146 w1157 w1164 w1172 w1184 w1196 w1205 w1213 w1229 w1237 w1247 w1256 w1265 w1274 w1282 w1297 w1302 w1313 w1323] -> w220
      tunnel: w217 -> [w914 w922 w934 w945 w955 w965 w976 w987 w997 w1006 w1017 w1030 w1044 w1052 w1073 w1085 w1090 w1099 w1112 w1120 w1136 w1156 w1167 w1174 w1186 w1198 w1207 w1215 w1231 w1240 w1250 w1259 w1268 w1277 w1285 w1300 w1305 w1316 w1326]
      tunnel: [w914 w922 w934 w945 w955 w965 w976 w987 w997 w1006 w1016 w1030 w1044 w1052 w1072 w1085 w1090 w1099 w1112 w1120 w1135 w1156 w1167 w1174 w1186 w1198 w1207 w1215 w1231 w1240 w1250 w1259 w1268 w1277 w1285 w1300 w1305 w1316 w1326] -> w216
      tunnel: w210 -> [w909 _ _ _ _ _ _ _ _ _ _ _ _ _ _ _ _ _ _ _ _ _ _ _ _ _ _ _ w1225 _ _ _ _ _ _ _ _ _ _]
      tunnel: w209 -> [_ _ _ _ _ _ _ _ _ _ _ _ _ _ _ _ _ _ _ _ _ _ _ _ _ _ w1199 _ w1227 w1236 _ _ _ _ _ _ _ _ _]
      tunnel: w208 -> [w913 w921 w933 w944 w954 w964 w975 w986 w995 w1003 w1015 w1029 w1037 w1049 w1064 w1082 w1089 w1098 w1109 w1117 w1141 w1154 w1166 w1171 w1183 w1195 w1201 w1212 w1222 w1239 w1249 w1258 w1267 w1276 w1284 w1299 w1304 w1315 w1325]
      tunnel: [w913 w921 w933 w944 w954 w964 w975 w986 w995 w1003 w1015 w1029 w1037 w1049 w1063 w1082 w1089 w1098 w1109 w1117 w1140 w1154 w1166 w1171 w1183 w1195 w1201 w1212 w1221 w1239 w1249 w1258 w1267 w1276 w1284 w1299 w1304 w1315 w1325] -> w207
      tunnel: w205 -> [w912 w920 w932 w943 w953 w963 w974 w985 w994 w1002 w1014 w1028 w1045 w1048 w1069 w1081 w1088 w1097 w1108 w1116 w1131 w1153 w1163 w1170 w1182 w1194 w1204 w1211 w1232 w1241 w1246 w1255 w1264 w1273 w1286 w1296 w1306 w1317 w1327]
      tunnel: [w912 w920 w932 w943 w953 w963 w974 w985 w994 w1002 w1014 w1028 w1045 w1048 w1068 w1081 w1088 w1097 w1108 w1116 w1130 w1153 w1163 w1170 w1182 w1194 w1204 w1211 w1232 w1241 w1246 w1255 w1264 w1273 w1286 w1295 w1306 w1317 w1327] -> w204
      tunnel: w202 -> [w911 w919 w927 w938 w948 w962 w969 w980 w993 w1001 w1008 w1021 w1040 w1047 w1059 w1080 w1087 w1096 w1107 w1115 w1127 w1152 w1160 w1169 w1181 w1193 w1203 w1210 w1233 w1242 w1245 w1252 w1261 w1270 w1287 w1290 w1307 w1318 w1328]
      tunnel: [w911 w919 w927 w938 w948 w962 w969 w980 w993 w1001 w1008 w1021 w1039 w1047 w1058 w1080 w1087 w1096 w1107 w1115 w1126 w1152 w1160 w1169 w1181 w1193 w1203 w1210 w1233 w1242 w1245 w1252 w1261 w1270 w1287 w1290 w1307 w1318 w1328] -> w201
      tunnel: w199 -> [w908 w918 w928 w939 w949 w958 w970 w981 w990 w1000 w1007 w1020 w1036 w1046 w1053 w1077 w1086 w1095 w1106 w1113 w1124 w1150 w1159 w1168 w1180 w1192 w1202 w1209 w1234 w1243 w1244 w1251 w1260 w1269 w1288 w1289 w1301 w1311 w1321]
      tunnel: [w908 w918 w928 w939 w949 w958 w970 w981 w990 w1000 w1007 w1020 w1036 w1046 w1053 w1077 w1086 w1095 w1106 w1113 w1123 w1150 w1159 w1168 w1180 w1192 w1202 w1209 w1234 w1243 w1244 w1251 w1260 w1269 w1288 w1289 w1301 w1309 w1320] -> w198
      tunnel: w196 -> [_ _ _ _ _ _ _ _ _ _ _ _ _ _ _ _ _ _ _ _ _ _ _ _ _ _ _ _ _ _ _ _ _ _ w1279 _ _ _ _]
      frame "Exit" {
        # ">>State Logic  >>"
        # ">>> Time cluster >>>"
        # ">>> Yaw >>>"
        # ">>> Stepper position >>>"
        # ">>> Encoders >>>"
        # ">>> Object detection >>>"
        # ">>> Ultrasonic Sensors Detect >>>"
        n60 = call "Imaq Dispose"("All Images? (No)"=TRUE, "Image"=w909) -> ()  [unwired: 4 in, 1 out]
      }
      frame "----Movement States----" {
        # ">>State Logic  >>"
        # ">>> Time cluster >>>"
        # ">>> Yaw >>>"
        # ">>> Stepper position >>>"
        # ">>> Encoders >>>"
        # ">>> Object detection >>>"
        # ">>> Ultrasonic Sensors Detect >>>"
      }
      frame "FORWARD" {
        # ">>> Time cluster >>>"
        # ">>> Yaw >>>"
        # ">>> Stepper position >>>"
        # ">>> Encoders >>>"
        # ">>> Object detection >>>"
        # ">>> Ultrasonic Sensors Detect >>>"
        n61 = Unbundle By Name(w927) -> ("Yaw"=w926:dbl)
        n62 = call "Motor Control NO PID AE Ver.vi"("Direction"=MOTOR_CONTROL_NO_PID_AE_DIRECTIONS_type_def."y-axis movement", "AE Mode"=MOTOR_CONTROL_NO_PID_AE_DATA_ENTRY_MODE_Type_def."Write to motors", "Speed"=0.5, "Yaw"=w926) -> ()  [unwired: 1 in, 2 out]
      }
      frame "LEFT" {
        # ">>State Logic  >>"
        # ">>> Time cluster >>>"
        # ">>> Yaw >>>"
        # ">>> Stepper position >>>"
        # ">>> Encoders >>>"
        # ">>> Object detection >>>"
        # ">>> Ultrasonic Sensors Detect >>>"
        n63 = Unbundle By Name(w938) -> ("Yaw"=w937:dbl)
        n64 = call "Motor Control NO PID AE Ver.vi"("Direction"=MOTOR_CONTROL_NO_PID_AE_DIRECTIONS_type_def."x-axis movement", "AE Mode"=MOTOR_CONTROL_NO_PID_AE_DATA_ENTRY_MODE_Type_def."Write to motors", "Speed"=-0.5, "Yaw"=w937) -> ()  [unwired: 1 in, 2 out]
      }
      frame "R-ACW" {
        n65 = call "Motor Control NO PID AE Ver.vi"("Direction"=MOTOR_CONTROL_NO_PID_AE_DIRECTIONS_type_def."Rotate", "AE Mode"=MOTOR_CONTROL_NO_PID_AE_DATA_ENTRY_MODE_Type_def."Write to motors", "Speed"=0.5) -> ()  [unwired: 2 in, 2 out]
      }
      frame "R-CW" {
        (unwired) -0.2 ("Speed")
        n66 = call "Motor Control NO PID AE Ver.vi"("Direction"=MOTOR_CONTROL_NO_PID_AE_DIRECTIONS_type_def."Rotate", "AE Mode"=MOTOR_CONTROL_NO_PID_AE_DATA_ENTRY_MODE_Type_def."Write to motors", "Speed"=-0.5) -> ()  [unwired: 2 in, 2 out]
      }
      frame "RIGHT" {
        n67 = Unbundle By Name(w969) -> ("Yaw"=w968:dbl)
        n68 = call "Motor Control NO PID AE Ver.vi"("Direction"=MOTOR_CONTROL_NO_PID_AE_DIRECTIONS_type_def."x-axis movement", "AE Mode"=MOTOR_CONTROL_NO_PID_AE_DATA_ENTRY_MODE_Type_def."Write to motors", "Speed"=-0.5, "Yaw"=w968) -> ()  [unwired: 1 in, 2 out]
      }
      frame "REVERSE" {
        n69 = Unbundle By Name(w980) -> ("Yaw"=w979:dbl)
        n70 = call "Motor Control NO PID AE Ver.vi"("Direction"=MOTOR_CONTROL_NO_PID_AE_DIRECTIONS_type_def."y-axis movement", "AE Mode"=MOTOR_CONTROL_NO_PID_AE_DATA_ENTRY_MODE_Type_def."Write to motors", "Speed"=-0.5, "Yaw"=w979) -> ()  [unwired: 1 in, 2 out]
      }
      frame "STOP" {
        n71 = Wait (ms)(milliseconds to wait=u32 500) -> ()  [unwired: 1 out]
        n72 = call "Motor Control NO PID AE Ver.vi"("Direction"=MOTOR_CONTROL_NO_PID_AE_DIRECTIONS_type_def."Stop", "AE Mode"=MOTOR_CONTROL_NO_PID_AE_DATA_ENTRY_MODE_Type_def."Write to motors") -> ()  [unwired: 3 in, 2 out]
      }
      frame "----SENSOR READING---- " {
      }
      frame "READ ENCODERS" {
        # ">>> Time cluster >>>"
        # ">>> Yaw >>>"
        # ">>> Stepper position >>>"
        # ">>> Object detection >>>"
        # ">>> Current encoder distance >>>"
        # ">>> Ultrasonic Sensors Detect >>>"
        n73 = call "Motor Control NO PID AE Ver.vi"("AE Mode"=MOTOR_CONTROL_NO_PID_AE_DATA_ENTRY_MODE_Type_def."Read from Encoders") -> ("Speed & distance"=w1012:T2)  [unwired: 4 in, 1 out]
        n74 = Unbundle By Name(w1012) -> ("xDistance"=w1011:dbl, "yDistance"=w1010:dbl, "wDistance"=w1009:dbl)
        n75 = Bundle By Name(cluster=w1017, "xDistance"=w1011, "yDistance"=w1010, "wDistance"=w1009) -> (w1016:T15)
      }
      frame "READ ULTRASONIC" {
        (unwired) navX_type_def."Read Values" ("Mode")
        (unwired) MOTOR_CONTROL_NO_PID_Type_Def."Latch" ("Direction")
        # ">>> Ultrasonic Sensors Detect >>>"
        # ">>> Object detection >>>"
        # ">>> Encoders >>>"
        # ">>> Stepper position >>>"
        # ">>> Yaw >>>"
        n76 = call "Arduino Interfacing VI.vi"("AE Mode"=Arduino_Interfacing."Read From Arduino") -> ("Arduino Data"=w1026:T4)  [unwired: 3 in, 1 out]
        n77 = Unbundle By Name(w1026) -> ("PING A"=w1025:u8, "PING B"=w1024:u8, "PING C"=w1023:u8, "PING D"=w1022:u8)
        n78 = Bundle By Name(cluster=w1032, "PING_A"=w1025, "PING_B"=w1024, "PING_C"=w1023, "PING_D"=w1022) -> (w1033:T14)
      }
      frame "READ YAW" {
        # ">>> Time cluster >>>"
        # ">>> Yaw >>>"
        # ">>> Ultrasonic Sensors Detect >>>"
        # ">>> Object detection >>>"
        # ">>> Encoders >>>"
        # ">>> Stepper position >>>"
        n79 = call "navX reading VI.vi"("Mode"=navX_type_def."Read Values") -> ("NavX Readings"=w1035:T3)  [unwired: 2 in, 3 out]
        n80 = Unbundle By Name(w1035) -> ("Heading"=w1034:dbl)
        n81 = Unbundle By Name(w1035) -> ("Yaw"=w1038:dbl)
        n82 = Bundle By Name(cluster=w1040, "Yaw"=w1038, "Compass"=w1034) -> (w1039:T10)
      }
      frame "----SYSTEM MODES----" {
        (unwired) I2C_MASTER_Type_Def."Last State" ("Arduino Mode")
        # ">>> Object detection >>>"
        # ">>> Yaw >>>"
        # ">>> Ultrasonic Sensors Detect >>>"
        # ">>> Encoders >>>"
        # ">>> Stepper position >>>"
      }
      frame "INIT" {
        w1070 = u8 0
        w1071 = 0.0
        # ">>> Time cluster >>>"
        # ">>> Object detection >>>"
        # ">>> Yaw >>>"
        # ">>> Ultrasonic Sensors Detect >>>"
        # ">>> Encoders >>>"
        # ">>> Stepper position >>>"
        # ">>State Logic  >>"
        n83 = call "Arduino Interfacing VI.vi"("AE Mode"=Arduino_Interfacing."Initialize") -> ()  [unwired: 3 in, 2 out]
        n84 = call "FGV Bool.vi"("Init/Read/Write State"=States_for_Action_Engine."Initialize") -> ()  [unwired: 2 in, 2 out]
        n85 = call "Motor Control NO PID AE Ver.vi"("AE Mode"=MOTOR_CONTROL_NO_PID_AE_DATA_ENTRY_MODE_Type_def."Initialize") -> ()  [unwired: 4 in, 2 out]
        n86 = call "Elasped Timer.vi"("Action"=Control."Initialize") -> ()  [unwired: 7 in, 4 out]
        n87 = Bundle By Name(cluster=w1064, "Recognized Object"=FALSE, "Object X coordinate"=0.0, "Object Y coordinate"=0.0) -> (w1063:T13)
        n88 = Bundle By Name(cluster=w1069, "y Stepper Position"=u8 0, "z Stepper Position"=u8 0) -> (w1068:T11)
        n89 = Bundle By Name(cluster=w1073, "xDistance"=w1071, "yDistance"=w1071, "wDistance"=w1071) -> (w1072:T15)
        n90 = Bundle By Name(cluster=w1075, "PING_A"=w1070, "PING_B"=w1070, "PING_C"=w1070, "PING_D"=w1070) -> (w1076:T14)
        n91 = Bundle By Name(cluster=w1059, "Yaw"=0.0) -> (w1058:T10)
      }
      frame "ARDUINO - ULTRASONIC" {
        # ">>> Object detection >>>"
        # ">>> Yaw >>>"
        # ">>> Ultrasonic Sensors Detect >>>"
        # ">>> Encoders >>>"
        # ">>> Stepper position >>>"
        # ">>State Logic  >>"
        n92 = call "Arduino Interfacing VI.vi"("Data to Write"=I2C_MASTER_WRITE_NEW_Type_Def."Ultrasonic sensors", "AE Mode"=Arduino_Interfacing."Write to Arduino") -> ()  [unwired: 2 in, 2 out]
      }
      frame "NAVX CALIBRATE" {
        # ">>> Object detection >>>"
        # ">>> Yaw >>>"
        # ">>> Ultrasonic Sensors Detect >>>"
        # ">>> Encoders >>>"
        # ">>> Stepper position >>>"
        # ">>State Logic  >>"
        # "Adds a 15 second delay to the startup process \nfor the NavX to calibrate"
        n93 = Wait (ms)(milliseconds to wait=u32 5000) -> ()  [unwired: 1 out]
      }
      frame "NO ACTION", Default {
        (unwired) u8 0 ("y Stepper value")
        (unwired) TRUE ("Latch")
        (unwired) navX_type_def."Read Values" ("Mode")
        (unwired) MOTOR_CONTROL_NO_PID_Type_Def."Latch" ("Direction")
        # ">>> Object detection >>>"
        # ">>> Yaw >>>"
        # ">>> Ultrasonic Sensors Detect >>>"
        # ">>> Encoders >>>"
        # ">>> Stepper position >>>"
        # ">>State Logic  >>"
        n94 = case shown="4" w1100 {
          tunnel: [0 100] -> w1102
          frame 1, Default {
          }
          frame 4 {
          }
        }
      }
      frame "----RESET CASES----" {
        (unwired) I2C_MASTER_Type_Def."Last State" ("Arduino Mode")
        # ">>> Object detection >>>"
        # ">>> Yaw >>>"
        # ">>> Ultrasonic Sensors Detect >>>"
        # ">>> Encoders >>>"
        # ">>> Stepper position >>>"
        # ">>State Logic  >>"
      }
      frame "RESET ENCODERS" {
        # ">>> Object detection >>>"
        # ">>> Yaw >>>"
        # ">>> Ultrasonic Sensors Detect >>>"
        # ">>> Encoders >>>"
        # ">>> Stepper position >>>"
        # ">>State Logic  >>"
        n95 = call "Motor Control NO PID AE Ver.vi"("AE Mode"=MOTOR_CONTROL_NO_PID_AE_DATA_ENTRY_MODE_Type_def."Reset Encoders") -> ()  [unwired: 4 in, 2 out]
      }
      frame "RESET FLAGS" {
        (unwired) I2C_MASTER_Type_Def."Last State" ("Arduino Mode")
        # "Resets any software variables\nand/or non-critical states"
        n96 = Wait (ms)(milliseconds to wait=u32 20) -> ()  [unwired: 1 out]
        n97 = Bundle By Name(cluster=w1124, "Time up flag"=FALSE, "SET TIME TO CHECK"=0.0) -> (w1123:T9)
        n98 = Bundle By Name(cluster=w1141, "Recognized Object"=FALSE, "Object X coordinate"=0.0, "Object Y coordinate"=0.0) -> (w1140:T13)
        n99 = Bundle By Name(cluster=w1131, "y Stepper Position"=u8 0, "z Stepper Position"=u8 0) -> (w1130:T11)
        n100 = Bundle By Name(cluster=w1136, "xDistance"=0.0, "yDistance"=0.0, "wDistance"=0.0) -> (w1135:T15)
        n101 = Bundle By Name(cluster=w1148, "PING_A"=u8 0, "PING_B"=u8 0, "PING_C"=u8 0, "PING_D"=u8 0) -> (w1147:T14)
        n102 = Bundle By Name(cluster=w1127, "Yaw"=0.0) -> (w1126:T10)
      }
      frame "RESET YAW" {
        n103 = Wait (ms)(milliseconds to wait=u32 100) -> ()  [unwired: 1 out]
        n104 = call "navX reading VI.vi"("Mode"=navX_type_def."Zero Yaw") -> ()  [unwired: 2 in, 4 out]
      }
      frame "RESET ARM" {
        n105 = call "Arduino Interfacing VI.vi"("Data to Write"=I2C_MASTER_WRITE_NEW_Type_Def."Soft Reset", "AE Mode"=Arduino_Interfacing."Write to Arduino") -> ()  [unwired: 2 in, 2 out]
      }
      frame "--------CAM STATES-------" {
      }
      frame "OPEN LOG CAM" {
        n106 = call "Webcam AE.vi"("Session In"=T30 "cam0", "Camera states"=Webcam_AE."Initialize Camera") -> ("error out"=w1177:errorcluster, "Session Out"=w1176:T30)  [unwired: 1 in, 1 out]
        n107 = call "Webcam AE.vi"("error in (no error)"=w1177, "Session In"=w1176, "Camera states"=Webcam_AE."Open Camera") -> ()  [unwired: 3 out]
      }
      frame "OPEN LIFE CAM" {
        n108 = call "Webcam AE.vi"("Session In"=T30 "cam1", "Camera states"=Webcam_AE."Initialize Camera") -> ("error out"=w1189:errorcluster, "Session Out"=w1188:T30)  [unwired: 1 in, 1 out]
        n109 = call "Webcam AE.vi"("error in (no error)"=w1189, "Session In"=w1188, "Camera states"=Webcam_AE."Open Camera") -> ()  [unwired: 3 out]
      }
      frame "CAM ACQ" {
        # ">>State Logic  >>"
        # ">>> Time cluster >>>"
        # ">>> Yaw >>>"
        # ">>> Stepper position >>>"
        # ">>> Encoders >>>"
        # ">>> Object detection >>>"
        # ">>> Ultrasonic Sensors Detect >>>"
        n110 = call "Webcam AE.vi"("error in (no error)"=w1199, "Camera states"=Webcam_AE."Continuous Acquisition") -> ()  [unwired: 1 in, 3 out]
      }
      frame "CAM CLOSE" {
        # ">>State Logic  >>"
        # ">>> Time cluster >>>"
        # ">>> Yaw >>>"
        # ">>> Stepper position >>>"
        # ">>> Encoders >>>"
        # ">>> Object detection >>>"
        # ">>> Ultrasonic Sensors Detect >>>"
        n111 = call "Webcam AE.vi"("Camera states"=Webcam_AE."Close Camera") -> ()  [unwired: 2 in, 3 out]
      }
      frame "PROCESS IMAGE" {
        # ">>State Logic  >>"
        # ">>> Time cluster >>>"
        # ">>> Yaw >>>"
        # ">>> Stepper position >>>"
        # ">>> Encoders >>>"
        # ">>> Object detection >>>"
        # ">>> Ultrasonic Sensors Detect >>>"
        n112 = call "Webcam AE.vi"("error in (no error)"=w1227, "Camera states"=Webcam_AE."Retrieve Image") -> ("error out"=w1223:errorcluster, "Image Out"=w1226:T23)  [unwired: 1 in, 1 out]
        n113 = call "Object Detection SubVI.vi"("Error In"=w1223, "Mode"="Object recognition mode", "Image Dest"=w1225, "Image in"=w1226) -> ("Object Center Coordinates"=w1220:cluster{"x":sgl, "y":sgl}, "Object detection cluster"=w1216:T1)  [unwired: 2 out]
        "Object detection cluster" <- w1216
        "Object Center Coordinates" <- w1220
        n114 = Unbundle By Name(w1216) -> ("Object detected?"=w1217:bool)
        n115 = Unbundle By Name(w1220) -> ("x"=w1219:sgl, "y"=w1218:sgl)
        n116 = Bundle By Name(cluster=w1222, "Recognized Object"=w1217, "Object X coordinate"=w1219, "Object Y coordinate"=w1218) -> (w1221:T13)
      }
      frame "DISPOSE BUFFERS" {
        # ">>State Logic  >>"
        # ">>> Time cluster >>>"
        # ">>> Yaw >>>"
        # ">>> Stepper position >>>"
        # ">>> Encoders >>>"
        # ">>> Object detection >>>"
        # ">>> Ultrasonic Sensors Detect >>>"
        n117 = call "Webcam AE.vi"("error in (no error)"=w1236, "Camera states"=Webcam_AE."Dispose Image Buffers") -> ()  [unwired: 1 in, 3 out]
      }
      frame "-----ARM ACTIONS-----" {
      }
      frame "CLOSE CLAW" {
        n118 = call "Arduino Interfacing VI.vi"("Data to Write"=I2C_MASTER_WRITE_NEW_Type_Def."Close Claw", "AE Mode"=Arduino_Interfacing."Write to Arduino") -> ()  [unwired: 2 in, 2 out]
      }
      frame "OPEN CLAW" {
        n119 = call "Arduino Interfacing VI.vi"("Data to Write"=I2C_MASTER_WRITE_NEW_Type_Def."Open Claw", "AE Mode"=Arduino_Interfacing."Write to Arduino") -> ()  [unwired: 2 in, 2 out]
      }
      frame "Z STEPPER CAM HEIGHT" {
        n120 = call "Arduino Interfacing VI.vi"("Data to Write"=I2C_MASTER_WRITE_NEW_Type_Def."zStepper 8k", "AE Mode"=Arduino_Interfacing."Write to Arduino") -> ()  [unwired: 2 in, 2 out]
      }
      frame "Y STEPPER CONTROL" {
        # ">>> yStepper command>>>"
        # ">>> Time cluster >>>"
        # ">>> Yaw >>>"
        # ">>> Stepper position >>>"
        # ">>> Encoders >>>"
        # ">>> Object detection >>>"
        # ">>> Ultrasonic Sensors Detect >>>"
        n121 = Unbundle By Name(w1279) -> ("yStepper desired"=w1278:u8)
        n122 = call "Arduino Interfacing VI.vi"("y Stepper value"=w1278, "Data to Write"=I2C_MASTER_WRITE_NEW_Type_Def."yStepper control", "AE Mode"=Arduino_Interfacing."Write to Arduino") -> ()  [unwired: 1 in, 2 out]
      }
      frame "READ STEPPER VALUES" {
        # ">>State Logic  >>"
        # ">>> Time cluster >>>"
        # ">>> Yaw >>>"
        # ">>> Stepper position >>>"
        # ">>> Encoders >>>"
        # ">>> Object detection >>>"
        # ">>> Ultrasonic Sensors Detect >>>"
        n123 = call "Arduino Interfacing VI.vi"("AE Mode"=Arduino_Interfacing."Read From Arduino") -> ("Arduino Data"=w1293:T4)  [unwired: 3 in, 1 out]
        n124 = Unbundle By Name(w1293) -> ("y Stepper Position"=w1292:u8, "z Stepper Position"=w1291:u8)
        n125 = Bundle By Name(cluster=w1296, "y Stepper Position"=w1292, "z Stepper Position"=w1291) -> (w1295:T11)
      }
      frame " -----TIMING-----" {
        # ">>State Logic  >>"
        # ">>> Time cluster >>>"
        # ">>> Yaw >>>"
        # ">>> Stepper position >>>"
        # ">>> Encoders >>>"
        # ">>> Object detection >>>"
        # ">>> Ultrasonic Sensors Detect >>>"
      }
      frame "SET TIMER" {
        # ">>State Logic  >>"
        # ">>> Time cluster >>>"
        # ">>> Yaw >>>"
        # ">>> Stepper position >>>"
        # ">>> Encoders >>>"
        # ">>> Object detection >>>"
        # ">>> Ultrasonic Sensors Detect >>>"
        n126 = call "Elasped Timer.vi"("Time Setting"=5.0, "Action"=Control."Initialize") -> ()  [unwired: 6 in, 4 out]
        n127 = Bundle By Name(cluster=w1311, "Time up flag"=FALSE) -> (w1309:T9)
      }
      frame "START TIMER" {
        # ">>State Logic  >>"
        # ">>> Time cluster >>>"
        # ">>> Yaw >>>"
        # ">>> Stepper position >>>"
        # ">>> Encoders >>>"
        # ">>> Object detection >>>"
        # ">>> Ultrasonic Sensors Detect >>>"
        n128 = call "Elasped Timer.vi"("Action"=Control."Start") -> ("Time Out?!"=w1319:bool)  [unwired: 7 in, 3 out]
        n129 = Bundle By Name(cluster=w1321, "Time up flag"=w1319) -> (w1320:T9)
      }
    }
    "State Logic" <- w220
    n130 = local read "TASK ENABLE"() -> (w214:bool)
    n131 = Not(x=w214) -> (.not. x?=w213:bool)
    n132 = case shown="True" w221 {
      tunnel: w225 -> [w248 w278]
      tunnel: w229 -> [w244 w280]
      tunnel: [w248 w278] -> w234
      tunnel: [w244 w281] -> w233
      tunnel: w230 -> [_ w276]
      tunnel: w232 -> [_ w277]
      tunnel: w227 -> [w247 w283]
      tunnel: [w247 w283] -> w226
      tunnel: "STOP TASK" -> [_ w266]
      tunnel: w220 -> [w246 w282]
      tunnel: [w246 w279] -> w219
      tunnel: w216 -> [w245 w272]
      tunnel: [w245 w272] -> w215
      tunnel: w213 -> [_ w267]
      tunnel: [w243 w264] -> w212
      tunnel: w211 -> [w243 w263]
      tunnel: w207 -> [w242 w260]
      tunnel: [w242 w260] -> w206
      tunnel: w204 -> [w241 w256]
      tunnel: [w241 w256] -> w203
      tunnel: w201 -> [w240 w254]
      tunnel: [w240 w254] -> w200
      tunnel: w198 -> [w239 w252]
      tunnel: [w239 w252] -> w197
      tunnel: w196 -> [w238 w251]
      tunnel: [w238 w250] -> w195
      frame False {
        # ">>> yStepper command>>>"
        # ">>> Time cluster >>>"
        # ">>> Yaw >>>"
        # ">>> Stepper position >>>"
        # ">>> Encoders >>>"
        # ">>> Object detection >>>"
        # ">>> Ultrasonic Sensors Detect >>>"
        # ">>> Time cluster >>>"
        # ">>> Yaw >>>"
        # ">>> Stepper position >>>"
        # ">>> Encoders >>>"
        # ">>> Object detection >>>"
        # ">>> Ultrasonic Sensors Detect >>>"
      }
      frame True {
        # ">>State Logic Queue Reference >>"
        # ">>Timeout>>"
        # ">>> yStepper command>>>"
        # ">>> Time cluster >>>"
        # ">>> Object detection >>>"
        # ">>> Yaw >>>"
        # ">>> Ultrasonic Sensors Detect >>>"
        # ">>> Encoders >>>"
        # ">>> Stepper position >>>"
        # ">>State Logic  >>"
        # ">>True Stop Next State >>"
        # ">>Action Queue>>"
        # ">> Manual override >>"
        # ">>> Time cluster >>>"
        # ">>> Yaw >>>"
        # ">>> Stepper position >>>"
        # ">>> Encoders >>>"
        # ">>> Object detection >>>"
        # ">>> Ultrasonic Sensors Detect >>>"
        # ">>Action Queue>>"
        # ">>State Logic Queue Reference >>"
        n133 = Or(x=w266, y=w267) -> (x .or. y?=w265:bool)
        n134 = Unbundle By Name(w254) -> ("Yaw"=w255:dbl, "Compass"=w249:dbl)
        n135 = Unbundle By Name(w252) -> ("Time up flag"=w253:bool)
        "Time up flag" <- w253
        n136 = Unbundle By Name(w256) -> ("y Stepper Position"=w258:u8, "z Stepper Position"=w257:u8)
        n137 = Unbundle By Name(w272) -> ("xDistance"=w269:dbl, "yDistance"=w270:dbl, "wDistance"=w271:dbl)
        n138 = Unbundle By Name(w260) -> ("Recognized Object"=w259:bool, "Object X coordinate"=w262:dbl, "Object Y coordinate"=w261:dbl)
        n139 = Unbundle By Name(w283) -> ("PING_A"=w275:u8, "PING_B"=w274:u8, "PING_C"=w273:u8, "PING_D"=w268:u8)
        n140 = case shown="15" w282 {
          tunnel: [w286 w290 w302 w310 w370 w383 w420 w467 w512 w570 w608 w663 w702 w744 w794 w837 w879] -> w281
          tunnel: w280 -> [w286 w293 w303 w313 w372 w384 w421 w468 w518 w563 w612 w653 w705 w750 w793 w832 w870]
          tunnel: [State_Type_Definitions."Idle" ("Enum") State_Type_Definitions."Idle" ("Enum") w298 w312 State_Type_Definitions."Shutdown" ("Enum") w385 w423 w466 w513 w569 w609 w662 w703 w751 w795 w838 w871] -> w279
          tunnel: w278 -> [_ _ w301 w316 _ w390 w433 w475 w517 w567 w613 w660 w699 w749 w791 w835 w878]
          tunnel: w277 -> [_ _ _ w315 _ w389 w432 w474 w516 w566 w605 w659 w698 w748 w790 w834 w876]
          tunnel: w276 -> [_ _ w300 w311 _ w388 w431 w473 w515 w565 w604 w661 w700 w747 w789 w833 w877]
          tunnel: w265 -> [_ _ _ _ _ w382 w422 w470 w511 w568 w610 w654 w706 w745 w792 w836 w874]
          tunnel: w275 -> [_ _ _ _ _ _ _ _ _ _ _ _ _ _ _ _ _]
          tunnel: w274 -> [_ _ _ _ _ _ w429 _ w509 w558 w615 _ _ _ _ _ _]
          tunnel: w273 -> [_ _ _ _ _ _ w428 _ w510 w559 w614 _ _ _ _ _ _]
          tunnel: w271 -> [_ _ _ _ _ _ _ w472 _ _ _ _ _ _ _ _ _]
          tunnel: w270 -> [_ _ _ _ _ w381 _ _ _ _ _ _ _ _ _ _ _]
          tunnel: w269 -> [_ _ _ _ _ _ _ _ _ w554 _ _ _ _ _ _ _]
          tunnel: w268 -> [_ _ _ _ _ _ _ _ _ _ _ _ _ _ _ _ _]
          tunnel: [State_Type_Definitions."Idle" ("Enum") State_Type_Definitions."Idle" ("Enum") State_Type_Definitions."Idle" ("Enum") State_Type_Definitions."Idle" ("Enum") State_Type_Definitions."Shutdown" ("Enum") w378 w419 w463 w504 w553 w607 w664 w704 w743 w796 w839 w872] -> w264
          tunnel: w263 -> [_ _ w298 _ _ _ _ _ _ _ _ _ _ _ _ _ _]
          tunnel: w259 -> [_ _ _ _ _ _ _ _ _ _ _ _ _ _ _ _ w873]
          tunnel: w262 -> [_ _ _ _ _ _ _ _ _ _ _ _ _ _ _ _ _]
          tunnel: w261 -> [_ _ _ _ _ _ _ _ _ _ _ _ _ w742 w781 _ _]
          tunnel: w258 -> [_ _ _ _ _ _ _ _ _ _ _ _ _ _ w784 _ _]
          tunnel: w257 -> [_ _ _ _ _ _ _ _ _ _ _ w657 _ _ _ w831 _]
          tunnel: w255 -> [_ _ _ _ _ _ _ _ _ _ _ _ _ _ _ _ _]
          tunnel: w253 -> [_ _ _ _ _ _ _ _ _ _ _ _ w701 _ _ _ _]
          tunnel: w251 -> [w284 w288 w297 w308 w368 w377 w418 w462 w503 w551 w603 w652 w696 w738 w787 w828 w869]
          tunnel: [w284 w288 w297 w308 w368 w377 w418 w462 w503 w551 w603 w652 w696 w738 w786 w828 w869] -> w250
          tunnel: w249 -> [_ _ _ _ _ _ _ _ _ _ _ _ _ _ _ _ _]
          frame 0 {
            # ">>> yStepper command>>>"
          }
          frame 1 {
            # ">>> yStepper command>>>"
            n141 = for {
              shift-right: [w296] -> w290
              shift-left: w293 -> [w295]
              tunnel: string[] ["INIT", "RESET ARM", "RESET FLAGS", "RESET YAW", "NAVX CALIBRATE"] -> [w294] mode=indexing
              n142 = Enqueue Element(queue=w295, element=w294) -> (queue out=w296:refnum<queue>)  [unwired: 2 in, 2 out]
            }
          }
          frame 3 {
            # ">>> yStepper command>>>"
            n143 = Flush Queue(queue=w301, error in (no error)=w300) -> ()  [unwired: 3 out]
            n144 = for {
              shift-right: [w307] -> w302
              shift-left: w303 -> [w306]
              tunnel: string[] ["STOP", "RESET ENCODERS", "RESET YAW", "RESET ARM", "RESET FLAGS", "DISPOSE BUFFERS", "CAM CLOSE"] -> [w305] mode=indexing
              n145 = Enqueue Element(queue=w306, element=w305) -> (queue out=w307:refnum<queue>)  [unwired: 2 in, 2 out]
            }
          }
          frame 4, Default {
            (unwired) TRUE ("Green LED")
            # ">>> yStepper command>>>"
            n146 = Dequeue Element(queue=w316, timeout in ms (-1)=w315, error in (no error)=w311) -> (element=w314:T7)  [unwired: 3 out]
            n147 = case shown="\"Start Task 5\"" w314 {
              tunnel: [w318 w325 w332 w339 w346 w353 w360 w362] -> w310
              tunnel: w313 -> [w319 w326 w333 w340 w347 w354 w360 w363]
              tunnel: [State_Type_Definitions."Task 1" ("Enum") State_Type_Definitions."Task 2" ("Enum") State_Type_Definitions."Task 3" ("Enum") State_Type_Definitions."Task 4_A" ("Enum") State_Type_Definitions."Task 5_A" ("Enum") State_Type_Definitions."Task 6_A" ("Enum") State_Type_Definitions."Idle" ("Enum") State_Type_Definitions."Shutdown" ("Enum")] -> w312
              frame "Start Task 1" {
                n148 = for {
                  shift-right: [w323] -> w318
                  shift-left: w319 -> [w322]
                  tunnel: string[] ["RESET ENCODERS", "RESET YAW", "FORWARD", "READ ENCODERS"] -> [w321] mode=indexing
                  n149 = Enqueue Element(queue=w322, element=w321) -> (queue out=w323:refnum<queue>)  [unwired: 2 in, 2 out]
                }
              }
              frame "Start Task 2" {
                n150 = for {
                  shift-right: [w330] -> w325
                  shift-left: w326 -> [w329]
                  tunnel: string[] ["RESET ENCODERS", "RESET YAW", "READ ULTRASONIC", "ARDUINO - ULTRASONIC"] -> [w328] mode=indexing
                  n151 = Enqueue Element(queue=w329, element=w328) -> (queue out=w330:refnum<queue>)  [unwired: 2 in, 2 out]
                }
              }
              frame "Start Task 3" {
                n152 = for {
                  shift-right: [w337] -> w332
                  shift-left: w333 -> [w336]
                  tunnel: string[] ["RESET ENCODERS", "READ ENCODERS", "R-ACW"] -> [w335] mode=indexing
                  n153 = Enqueue Element(queue=w336, element=w335) -> (queue out=w337:refnum<queue>)  [unwired: 2 in, 2 out]
                }
              }
              frame "Start Task 4" {
                n154 = for {
                  shift-right: [w344] -> w339
                  shift-left: w340 -> [w343]
                  tunnel: string[] ["STOP", "RESET YAW", "RESET ENCODERS", "READ ULTRASONIC", "ARDUINO - ULTRASONIC", ""] -> [w342] mode=indexing
                  n155 = Enqueue Element(queue=w343, element=w342) -> (queue out=w344:refnum<queue>)  [unwired: 2 in, 2 out]
                }
              }
              frame "Start Task 5" {
                n156 = for {
                  shift-right: [w351] -> w346
                  shift-left: w347 -> [w350]
                  tunnel: string[] ["RESET YAW", "RESET ENCODERS", "READ STEPPER VALUES", "Z STEPPER CAM HEIGHT", "", ""] -> [w349] mode=indexing
                  n157 = Enqueue Element(queue=w350, element=w349) -> (queue out=w351:refnum<queue>)  [unwired: 2 in, 2 out]
                }
              }
              frame "Start Task 6" {
                n158 = for {
                  shift-right: [w358] -> w353
                  shift-left: w354 -> [w357]
                  tunnel: string[] ["Z STEPPER CAM HEIGHT ", "READ STEPPER VALUES", "OPEN LOG CAM", "", "", ""] -> [w356] mode=indexing
                  n159 = Enqueue Element(queue=w357, element=w356) -> (queue out=w358:refnum<queue>)  [unwired: 2 in, 2 out]
                }
              }
              frame "None", Default {
              }
              frame "Exit" {
                n160 = for {
                  shift-right: [w367] -> w362
                  shift-left: w363 -> [w366]
                  tunnel: string[] ["STOP", "RESET ENCODERS", "RESET YAW", "EXIT"] -> [w365] mode=indexing
                  n161 = Enqueue Element(queue=w366, element=w365) -> (queue out=w367:refnum<queue>)  [unwired: 2 in, 2 out]
                }
              }
            }
          }
          frame 5 {
            # ">>> yStepper command>>>"
            n162 = for {
              shift-right: [w376] -> w370
              shift-left: w372 -> [w375]
              tunnel: string[] ["INIT", "RESET ENCODERS", "RESET FLAGS", "EXIT"] -> [w374] mode=indexing
              n163 = Enqueue Element(queue=w375, element=w374) -> (queue out=w376:refnum<queue>)  [unwired: 2 in, 2 out]
            }
          }
          frame 6 {
            # ">>> yStepper command>>>"
            # "Use 250"
            n164 = Dequeue Element(queue=w390, timeout in ms (-1)=w389, error in (no error)=w388) -> (element=w387:T7)  [unwired: 3 out]
            n165 = Greater?(x=w381, y=10000.0) -> (0:w379:bool)
            n166 = Or(x=w379, y=w382) -> (x .or. y?=w386:bool)
            n167 = case shown="\"None\", Default" w387 {
              tunnel: w386 -> [w393 _]
              tunnel: [w397 State_Type_Definitions."True Stop" ("Enum")] -> w385
              tunnel: w384 -> [w394 w412]
              tunnel: [w392 w411] -> w383
              tunnel: [State_Type_Definitions."Idle" ("Enum") State_Type_Definitions."Shutdown" ("Enum")] -> w378
              frame "None", Default {
                n168 = case shown="True" w393 {
                  tunnel: w394 -> [w400 w406]
                  tunnel: [w399 w404] -> w392
                  frame False {
                    n169 = for {
                      shift-right: [w402] -> w399
                      shift-left: w400 -> [w403]
                      tunnel: string[] ["READ ENCODERS", "READ YAW", "FORWARD"] ("element") -> [w401] mode=indexing
                      n170 = Enqueue Element(queue=w403, element=w401) -> (queue out=w402:refnum<queue>)  [unwired: 2 in, 2 out]
                    }
                  }
                  frame True {
                    n171 = for {
                      shift-right: [w408] -> w404
                      shift-left: w406 -> [w409]
                      tunnel: string[] ["RESET YAW", "RESET ENCODERS", "STOP", ""] -> [w407] mode=indexing
                      n172 = Enqueue Element(queue=w409, element=w407) -> (queue out=w408:refnum<queue>)  [unwired: 2 in, 2 out]
                    }
                  }
                }
                n173 = Select(t=State_Type_Definitions."True Stop" ("Enum"), s=w393, f=State_Type_Definitions."Task 1" ("Enum")) -> (s? t:f=w397:u16)
              }
              frame "Exit" {
                n174 = for {
                  shift-right: [w416] -> w411
                  shift-left: w412 -> [w417]
                  tunnel: string[] ["STOP", "RESET ENCODERS", "RESET YAW", ""] -> [w415] mode=indexing
                  n175 = Enqueue Element(queue=w417, element=w415) -> (queue out=w416:refnum<queue>)  [unwired: 2 in, 2 out]
                }
              }
            }
          }
          frame 7 {
            w427 = u8 10 ("y")
            # ">>> yStepper command>>>"
            # ">>Object detected>>"
            n176 = Dequeue Element(queue=w433, timeout in ms (-1)=w432, error in (no error)=w431) -> (element=w430:T7)  [unwired: 3 out]
            n177 = Less?(x=w429, y=w427) -> (x < y?=w426:bool)
            n178 = Less?(x=w428, y=w427) -> (x < y?=w425:bool)
            n179 = Or(x=w426, y=w425) -> (x .or. y?=w424:bool)
            "Obstacle detected" <- w424
            n180 = case shown="\"None\", Default" w430 {
              tunnel: w424 -> [w437 _]
              tunnel: [w439 State_Type_Definitions."True Stop" ("Enum")] -> w423
              tunnel: w422 -> [w438 _]
              tunnel: w421 -> [w436 w456]
              tunnel: [w435 w457] -> w420
              tunnel: [State_Type_Definitions."Idle" ("Enum") State_Type_Definitions."Shutdown" ("Enum")] -> w419
              frame "None", Default {
                n181 = case shown="False" w437 {
                  tunnel: w436 -> [w443 w450]
                  tunnel: [w444 w449] -> w435
                  frame False {
                    n182 = for {
                      tunnel: string[] ["READ ULTRASONIC", "STOP"] ("element") -> [w445] mode=indexing
                      shift-right: [w447] -> w444
                      shift-left: w443 -> [w446]
                      n183 = Enqueue Element(queue=w446, element=w445) -> (queue out=w447:refnum<queue>)  [unwired: 2 in, 2 out]
                    }
                  }
                  frame True {
                    n184 = for {
                      shift-right: [w452] -> w449
                      shift-left: w450 -> [w453]
                      tunnel: string[] ["REVERSE", "READ ULTRASONIC"] -> [w451] mode=indexing
                      n185 = Enqueue Element(queue=w453, element=w451) -> (queue out=w452:refnum<queue>)  [unwired: 2 in, 2 out]
                    }
                  }
                }
                n186 = Select(t=State_Type_Definitions."True Stop" ("Enum"), s=w438, f=State_Type_Definitions."Task 2" ("Enum")) -> (s? t:f=w439:u16)
              }
              frame "Exit" {
                n187 = for {
                  shift-right: [w460] -> w457
                  shift-left: w456 -> [w461]
                  tunnel: string[] ["STOP", "RESET ENCODERS", "RESET YAW", "ARDUINO MODE 0"] -> [w459] mode=indexing
                  n188 = Enqueue Element(queue=w461, element=w459) -> (queue out=w460:refnum<queue>)  [unwired: 2 in, 2 out]
                }
              }
            }
          }
          frame 8 {
            # ">>> yStepper command>>>"
            n189 = Dequeue Element(queue=w475, timeout in ms (-1)=w474, error in (no error)=w473) -> (element=w464:T7)  [unwired: 3 out]
            n190 = Greater?(x=w472, y=150.0) -> (0:w469:bool)
            n191 = Or(x=w469, y=w470) -> (x .or. y?=w465:bool)
            n192 = case shown="\"Exit\"" w464 {
              tunnel: w465 -> [w478 _]
              tunnel: [w482 State_Type_Definitions."True Stop" ("Enum")] -> w466
              tunnel: w468 -> [w479 w498]
              tunnel: [w477 w497] -> w467
              tunnel: [State_Type_Definitions."Idle" ("Enum") State_Type_Definitions."Shutdown" ("Enum")] -> w463
              frame "None", Default {
                n193 = case shown="False" w478 {
                  tunnel: w479 -> [w485 w491]
                  tunnel: [w484 w489] -> w477
                  frame False {
                    n194 = for {
                      shift-right: [w487] -> w484
                      shift-left: w485 -> [w488]
                      tunnel: string[] ["READ ENCODERS", "R-ACW"] ("element") -> [w486] mode=indexing
                      n195 = Enqueue Element(queue=w488, element=w486) -> (queue out=w487:refnum<queue>)  [unwired: 2 in, 2 out]
                    }
                  }
                  frame True {
                    n196 = for {
                      shift-right: [w493] -> w489
                      shift-left: w491 -> [w494]
                      tunnel: string[] ["RESET YAW", "RESET ENCODERS", "STOP", "ARDUINO MODE 0"] -> [w492] mode=indexing
                      n197 = Enqueue Element(queue=w494, element=w492) -> (queue out=w493:refnum<queue>)  [unwired: 2 in, 2 out]
                    }
                  }
                }
                n198 = Select(t=State_Type_Definitions."True Stop" ("Enum"), s=w478, f=State_Type_Definitions."Task 3" ("Enum")) -> (s? t:f=w482:T6)
              }
              frame "Exit" {
                n199 = for {
                  shift-right: [w501] -> w497
                  shift-left: w498 -> [w502]
                  tunnel: string[] ["STOP", "RESET ENCODERS", "RESET YAW", ""] -> [w500] mode=indexing
                  n200 = Enqueue Element(queue=w502, element=w500) -> (queue out=w501:refnum<queue>)  [unwired: 2 in, 2 out]
                }
              }
            }
          }
          frame 9 {
            w508 = u8 20
            # ">>> yStepper command>>>"
            # ">> Outputs true if object detected >>"
            # ">> Manual override >>"
            n201 = Dequeue Element(queue=w517, timeout in ms (-1)=w516, error in (no error)=w515) -> (element=w514:T7)  [unwired: 3 out]
            n202 = Less?(x=w510, y=w508) -> (x < y?=w506:bool)
            n203 = Less?(x=w509, y=w508) -> (x < y?=w507:bool)
            n204 = And(x=w507, y=w506) -> (x .and. y?=w505:bool)
            "Obstacle detected?" <- w505
            n205 = case shown="\"None\", Default" w514 {
              tunnel: [w527 State_Type_Definitions."True Stop" ("Enum")] -> w513
              tunnel: [w525 w546] -> w512
              tunnel: w518 -> [w524 _]
              tunnel: w511 -> [w522 _]
              tunnel: w505 -> [w520 _]
              tunnel: [w519 State_Type_Definitions."Shutdown" ("Enum")] -> w504
              frame "None", Default {
                # ">> WIill proceed to part ii if not manual override >>"
                # ">>If ENABLE or Trigger is set to true>>"
                n206 = Or(x=w520, y=w522) -> (x .or. y?=w521:bool)
                n207 = case shown="False" w521 {
                  tunnel: [w534 w539] -> w525
                  tunnel: w524 -> [w532 w538]
                  frame False {
                    n208 = for {
                      shift-right: [w536] -> w534
                      shift-left: w532 -> [w537]
                      tunnel: string[] ["FORWARD", "ULTRASONIC READ", ""] ("element") -> [w535] mode=indexing
                      n209 = Enqueue Element(queue=w537, element=w535) -> (queue out=w536:refnum<queue>)  [unwired: 2 in, 2 out]
                    }
                  }
                  frame True {
                    n210 = for {
                      shift-right: [w542] -> w539
                      shift-left: w538 -> [w543]
                      tunnel: string[] ["STOP", "RESET ENCODERS", "RESET YAW", "ARDUINO MODE 0"] -> [w541] mode=indexing
                      n211 = Enqueue Element(queue=w543, element=w541) -> (queue out=w542:refnum<queue>)  [unwired: 2 in, 2 out]
                    }
                  }
                }
                n212 = case shown="False" w522 {
                  tunnel: [State_Type_Definitions."True Stop" ("Enum") State_Type_Definitions."True Stop" ("Enum")] -> w523
                  tunnel: [State_Type_Definitions."Task 4_B" ("Enum") State_Type_Definitions."Idle" ("Enum")] -> w519
                  frame False {
                  }
                  frame True {
                  }
                }
                n213 = Select(t=w523, s=w521, f=State_Type_Definitions."Task 4_A" ("Enum")) -> (s? t:f=w527:T6)
              }
              frame "Exit" {
                n214 = for {
                  shift-right: [w549] -> w546
                  shift-left: _ -> [w550]
                  tunnel: string[] ["STOP", "RESET ENCODERS", "RESET YAW", ""] -> [w548] mode=indexing
                  n215 = Enqueue Element(queue=w550, element=w548) -> (queue out=w549:refnum<queue>)  [unwired: 2 in, 2 out]
                }
              }
            }
          }
          frame 10 {
            w562 = 20
            # ">>> yStepper command>>>"
            # ">> Outputs true if 150 mm has been moved >>"
            # ">> Outputs true if sensor not obstructed>>"
            # ">> Manual override >>"
            n216 = Dequeue Element(queue=w567, timeout in ms (-1)=w566, error in (no error)=w565) -> (element=w564:T7)  [unwired: 3 out]
            n217 = Greater?(x=w559, y=w562) -> (0:w560:bool)
            n218 = Greater?(x=w558, y=w562) -> (0:w561:bool)
            n219 = Greater Or Equal?(x=w554, y=80.0) -> (x >= y?=w556:bool)
            n220 = And(x=w561, y=w560) -> (x .and. y?=w555:bool)
            n221 = And(x=w556, y=w555) -> (x .and. y?=w552:bool)
            n222 = case shown="\"None\", Default" w564 {
              tunnel: [w579 State_Type_Definitions."True Stop" ("Enum")] -> w569
              tunnel: [w577 w598] -> w570
              tunnel: w563 -> [w576 _]
              tunnel: w568 -> [w574 _]
              tunnel: w552 -> [w572 _]
              tunnel: [w571 State_Type_Definitions."Shutdown" ("Enum")] -> w553
              frame "None", Default {
                # ">> WIill proceed to part ii if not manual override >>"
                # ">>If ENABLE or Trigger is set to true>>"
                n223 = Or(x=w572, y=w574) -> (x .or. y?=w573:bool)
                n224 = case shown="False" w573 {
                  tunnel: [w586 w591] -> w577
                  tunnel: w576 -> [w584 w590]
                  frame False {
                    n225 = for {
                      shift-right: [w588] -> w586
                      shift-left: w584 -> [w589]
                      tunnel: string[] ["RIGHT", "ULTRASONIC READ", "READ ENCODERS"] ("element") -> [w587] mode=indexing
                      n226 = Enqueue Element(queue=w589, element=w587) -> (queue out=w588:refnum<queue>)  [unwired: 2 in, 2 out]
                    }
                  }
                  frame True {
                    n227 = for {
                      shift-right: [w594] -> w591
                      shift-left: w590 -> [w595]
                      tunnel: string[] ["STOP", "RESET ENCODERS", "RESET YAW", "ARDUINO MODE 0"] -> [w593] mode=indexing
                      n228 = Enqueue Element(queue=w595, element=w593) -> (queue out=w594:refnum<queue>)  [unwired: 2 in, 2 out]
                    }
                  }
                }
                n229 = case shown="True" w574 {
                  tunnel: [State_Type_Definitions."True Stop" ("Enum") State_Type_Definitions."True Stop" ("Enum")] -> w575
                  tunnel: [State_Type_Definitions."Task 4_C" ("Enum") State_Type_Definitions."Idle" ("Enum")] -> w571
                  frame False {
                  }
                  frame True {
                  }
                }
                n230 = Select(t=w575, s=w573, f=State_Type_Definitions."Task 4_B" ("Enum")) -> (s? t:f=w579:T6)
              }
              frame "Exit" {
                n231 = for {
                  shift-right: [w601] -> w598
                  shift-left: _ -> [w602]
                  tunnel: string[] ["STOP", "RESET ENCODERS", "RESET YAW", ""] -> [w600] mode=indexing
                  n232 = Enqueue Element(queue=w602, element=w600) -> (queue out=w601:refnum<queue>)  [unwired: 2 in, 2 out]
                }
              }
            }
          }
          frame 11 {
            w618 = u8 20
            # ">>> yStepper command>>>"
            # ">> Outputs true if object detected >>"
            # ">> Manual override >>"
            n233 = Dequeue Element(queue=w613, timeout in ms (-1)=w605, error in (no error)=w604) -> (element=w606:T7)  [unwired: 3 out]
            n234 = Less?(x=w614, y=w618) -> (x < y?=w616:bool)
            n235 = Less?(x=w615, y=w618) -> (x < y?=w617:bool)
            n236 = And(x=w617, y=w616) -> (x .and. y?=w611:bool)
            n237 = case shown="\"None\", Default" w606 {
              tunnel: [w627 State_Type_Definitions."True Stop" ("Enum")] -> w609
              tunnel: [w625 w647] -> w608
              tunnel: w612 -> [w624 w644]
              tunnel: w610 -> [w622 _]
              tunnel: w611 -> [w620 _]
              tunnel: [w619 State_Type_Definitions."Shutdown" ("Enum")] -> w607
              frame "None", Default {
                # ">> WIill proceed to part ii if not manual override >>"
                # ">>If ENABLE or Trigger is set to true>>"
                n238 = Or(x=w620, y=w622) -> (x .or. y?=w621:bool)
                n239 = case shown="False" w621 {
                  tunnel: [w634 w639] -> w625
                  tunnel: w624 -> [w632 w638]
                  frame False {
                    n240 = for {
                      shift-right: [w636] -> w634
                      shift-left: w632 -> [w637]
                      tunnel: string[] ["FORWARD", "ULTRASONIC READ", ""] ("element") -> [w635] mode=indexing
                      n241 = Enqueue Element(queue=w637, element=w635) -> (queue out=w636:refnum<queue>)  [unwired: 2 in, 2 out]
                    }
                  }
                  frame True {
                    n242 = for {
                      shift-right: [w642] -> w639
                      shift-left: w638 -> [w643]
                      tunnel: string[] ["STOP", "RESET ENCODERS", "RESET YAW", "ARDUINO MODE 0"] -> [w641] mode=indexing
                      n243 = Enqueue Element(queue=w643, element=w641) -> (queue out=w642:refnum<queue>)  [unwired: 2 in, 2 out]
                    }
                  }
                }
                n244 = case shown="True" w622 {
                  tunnel: [State_Type_Definitions."True Stop" ("Enum") State_Type_Definitions."True Stop" ("Enum")] -> w623
                  tunnel: [State_Type_Definitions."Idle" ("Enum") State_Type_Definitions."Idle" ("Enum")] -> w619
                  frame False {
                  }
                  frame True {
                  }
                }
                n245 = Select(t=w623, s=w621, f=State_Type_Definitions."Task 4_C" ("Enum")) -> (s? t:f=w627:T6)
              }
              frame "Exit" {
                n246 = for {
                  shift-right: [w650] -> w647
                  shift-left: w644 -> [w651]
                  tunnel: string[] ["STOP", "RESET ENCODERS", "RESET YAW", ""] -> [w649] mode=indexing
                  n247 = Enqueue Element(queue=w651, element=w649) -> (queue out=w650:refnum<queue>)  [unwired: 2 in, 2 out]
                }
              }
            }
          }
          frame 13 {
            # ">>> yStepper command>>>"
            # ">> Manual override >>"
            n248 = Dequeue Element(queue=w660, timeout in ms (-1)=w659, error in (no error)=w661) -> (element=w658:T7)  [unwired: 3 out]
            n249 = Equal?(x=w657, y=u8 80) -> (x = y?=w655:bool)
            n250 = case shown="\"None\", Default" w658 {
              tunnel: [w671 State_Type_Definitions."True Stop" ("Enum")] -> w662
              tunnel: [w674 w691] -> w663
              tunnel: [State_Type_Definitions."Idle" ("Enum") State_Type_Definitions."Shutdown" ("Enum")] -> w664
              tunnel: w655 -> [w670 _]
              tunnel: w654 -> [w669 _]
              tunnel: w653 -> [w665 w688]
              frame "None", Default {
                # "Stays in Task 5_A until stepper reaches desired \nheight"
                # "T: Go back to idle, F: Continue with task\""
                # ">> Manual override >>"
                n251 = case shown="True" w670 {
                  tunnel: [w678 w684] -> w674
                  tunnel: w665 -> [w676 w682]
                  frame False {
                    n252 = for {
                      tunnel: string[] ["Z STEPPER CAM HEIGHT", "READ STEPPER VALUES"] ("element") -> [w679] mode=indexing
                      shift-right: [w681] -> w678
                      shift-left: w676 -> [w680]
                      n253 = Enqueue Element(queue=w680, element=w679) -> (queue out=w681:refnum<queue>)  [unwired: 2 in, 2 out]
                    }
                  }
                  frame True {
                    n254 = for {
                      shift-right: [w686] -> w684
                      shift-left: w682 -> [w687]
                      tunnel: string[] ["OPEN LOG CAM", "SET TIMER", ""] -> [w685] mode=indexing
                      n255 = Enqueue Element(queue=w687, element=w685) -> (queue out=w686:refnum<queue>)  [unwired: 2 in, 2 out]
                    }
                  }
                }
                n256 = Or(x=w670, y=w669) -> (x .or. y?=w672:bool)
                n257 = Select(t=State_Type_Definitions."True Stop" ("Enum"), s=w669, f=State_Type_Definitions."Task 5 _B" ("Enum")) -> (s? t:f=w666:u16)
                n258 = Select(t=w666, s=w672, f=State_Type_Definitions."Task 5_A" ("Enum")) -> (s? t:f=w671:u16)
              }
              frame "Exit" {
                n259 = for {
                  shift-right: [w694] -> w691
                  shift-left: w688 -> [w695]
                  tunnel: string[] ["STOP", "RESET ENCODERS", "RESET YAW", "ARDUINO MODE 0"] -> [w693] mode=indexing
                  n260 = Enqueue Element(queue=w695, element=w693) -> (queue out=w694:refnum<queue>)  [unwired: 2 in, 2 out]
                }
              }
            }
          }
          frame 14 {
            # ">>> yStepper command>>>"
            n261 = Dequeue Element(queue=w699, timeout in ms (-1)=w698, error in (no error)=w700) -> (element=w697:T7)  [unwired: 3 out]
            n262 = case shown="\"None\", Default" w697 {
              tunnel: [w713 State_Type_Definitions."True Stop" ("Enum")] -> w703
              tunnel: [w716 w733] -> w702
              tunnel: [State_Type_Definitions."Idle" ("Enum") State_Type_Definitions."Shutdown" ("Enum")] -> w704
              tunnel: w701 -> [w712 _]
              tunnel: w706 -> [w711 _]
              tunnel: w705 -> [w707 w730]
              frame "None", Default {
                # "Stays in Task 5_B to capture image over 5 seconds"
                # "T: Go back to idle, F: Continue with task\""
                # ">> Manual override >>"
                n263 = case shown="False" w712 {
                  tunnel: [w720 w726] -> w716
                  tunnel: w707 -> [w718 w724]
                  frame False {
                    n264 = for {
                      tunnel: string[] ["CAM ACQ", "START TIMER"] ("element") -> [w721] mode=indexing
                      shift-right: [w723] -> w720
                      shift-left: w718 -> [w722]
                      n265 = Enqueue Element(queue=w722, element=w721) -> (queue out=w723:refnum<queue>)  [unwired: 2 in, 2 out]
                    }
                  }
                  frame True {
                    n266 = for {
                      shift-right: [w728] -> w726
                      shift-left: w724 -> [w729]
                      tunnel: string[] ["CAM CLOSE", "PROCESS IMAGE"] -> [w727] mode=indexing
                      n267 = Enqueue Element(queue=w729, element=w727) -> (queue out=w728:refnum<queue>)  [unwired: 2 in, 2 out]
                    }
                  }
                }
                n268 = Or(x=w712, y=w711) -> (x .or. y?=w714:bool)
                n269 = Select(t=State_Type_Definitions."True Stop" ("Enum"), s=w711, f=State_Type_Definitions."Task 5_C" ("Enum")) -> (s? t:f=w708:u16)
                n270 = Select(t=w708, s=w714, f=State_Type_Definitions."Task 5 _B" ("Enum")) -> (s? t:f=w713:u16)
              }
              frame "Exit" {
                n271 = for {
                  shift-right: [w736] -> w733
                  shift-left: w730 -> [w737]
                  tunnel: string[] ["STOP", "RESET ENCODERS", "RESET YAW", "ARDUINO MODE 0"] -> [w735] mode=indexing
                  n272 = Enqueue Element(queue=w737, element=w735) -> (queue out=w736:refnum<queue>)  [unwired: 2 in, 2 out]
                }
              }
            }
          }
          frame 15 {
            # ">>> yStepper command>>>"
            # ">> Checks if item is in range >>"
            # ">> Manual override >>"
            n273 = Dequeue Element(queue=w749, timeout in ms (-1)=w748, error in (no error)=w747) -> (element=w746:T7)  [unwired: 3 out]
            n274 = In Range and Coerce(upper limit=270.0, x=w742, lower limit=280.0) -> (In Range?=w739:bool)  [unwired: 1 out]
            n275 = case shown="\"None\", Default" w746 {
              tunnel: [w756 State_Type_Definitions."True Stop" ("Enum")] -> w751
              tunnel: [w759 w776] -> w744
              tunnel: [State_Type_Definitions."Idle" ("Enum") State_Type_Definitions."Shutdown" ("Enum")] -> w743
              tunnel: w739 -> [w755 _]
              tunnel: w745 -> [w754 _]
              tunnel: w750 -> [w753 w773]
              frame "None", Default {
                # ">> Is object in range? >>"
                # "Stays in Task 5_C until time is up and object is detected"
                # ">> Manual override >>"
                n276 = case shown="True" w755 {
                  tunnel: [w763 w769] -> w759
                  tunnel: w753 -> [w761 w767]
                  frame False {
                    n277 = for {
                      tunnel: string[] ["PROCESS IMAGE", ""] ("element") -> [w764] mode=indexing
                      shift-right: [w766] -> w763
                      shift-left: w761 -> [w765]
                      n278 = Enqueue Element(queue=w765, element=w764) -> (queue out=w766:refnum<queue>)  [unwired: 2 in, 2 out]
                    }
                  }
                  frame True {
                    n279 = for {
                      shift-right: [w771] -> w769
                      shift-left: w767 -> [w772]
                      tunnel: string[] ["CAM CLOSE", ""] -> [w770] mode=indexing
                      n280 = Enqueue Element(queue=w772, element=w770) -> (queue out=w771:refnum<queue>)  [unwired: 2 in, 2 out]
                    }
                  }
                }
                n281 = Or(x=w755, y=w754) -> (x .or. y?=w757:bool)
                n282 = Select(t=State_Type_Definitions."True Stop" ("Enum"), s=w757, f=State_Type_Definitions."Task 5_C_Error" ("Enum")) -> (s? t:f=w756:u16)
              }
              frame "Exit" {
                n283 = for {
                  shift-right: [w779] -> w776
                  shift-left: w773 -> [w780]
                  tunnel: string[] ["STOP", "RESET ENCODERS", "RESET YAW", "ARDUINO MODE 0"] -> [w778] mode=indexing
                  n284 = Enqueue Element(queue=w780, element=w778) -> (queue out=w779:refnum<queue>)  [unwired: 2 in, 2 out]
                }
              }
            }
          }
          frame 15 {
            # ">>> yStepper command>>>"
            # ">> Checks if yStepper has reached target>>"
            n285 = Dequeue Element(queue=w791, timeout in ms (-1)=w790, error in (no error)=w789) -> (element=w788:T7)  [unwired: 3 out]
            n286 = formula code="if (pos < 260)\ny = 25;\n\nelse if (pos >= 260 && pos < 280)\ny = 15;\n\nelse if (pos >= 280 && pos <= 300)\ny =10;\n\nelse if (pos > 300)\ny = 5;"("pos"=w781) -> ("y"=w785:dbl)
            n287 = To Unsigned Byte Integer(number=w785) -> (unsigned 8bit integer=w783:u8)
            n288 = Equal?(x=w784, y=w783) -> (x = y?=w782:bool)
            n289 = case shown="\"None\", Default" w788 {
              tunnel: [w803 State_Type_Definitions."True Stop" ("Enum")] -> w795
              tunnel: [w806 w823] -> w794
              tunnel: [State_Type_Definitions."Idle" ("Enum") State_Type_Definitions."Shutdown" ("Enum")] -> w796
              tunnel: w792 -> [w802 _]
              tunnel: w793 -> [w798 w820]
              tunnel: w782 -> [w797 _]
              frame "None", Default {
                # ">> T: Breaks out of state loop; F: Stays in loop>>"
                # ">> Manual override >>"
                # ">> Checks if yStepper has reached target>>"
                # "Stays in Task 5_C until time is up and object is detected"
                # "T: Go back to idle, F: Continue with task\""
                # ">> Manual override >>"
                n290 = case shown="True" w797 {
                  tunnel: [w810 w816] -> w806
                  tunnel: w798 -> [w808 w814]
                  frame False {
                    n291 = for {
                      tunnel: string[] ["Y STEPPER CONTROL", "READ STEPPER VALUES", ""] ("element") -> [w811] mode=indexing
                      shift-right: [w813] -> w810
                      shift-left: w808 -> [w812]
                      n292 = Enqueue Element(queue=w812, element=w811) -> (queue out=w813:refnum<queue>)  [unwired: 2 in, 2 out]
                    }
                  }
                  frame True {
                    n293 = for {
                      shift-right: [w818] -> w816
                      shift-left: w814 -> [w819]
                      tunnel: string[] ["OPEN LOG CAM", "CAM ACQ", "SET TIMER"] -> [w817] mode=indexing
                      n294 = Enqueue Element(queue=w819, element=w817) -> (queue out=w818:refnum<queue>)  [unwired: 2 in, 2 out]
                    }
                  }
                }
                n295 = Or(x=w797, y=w802) -> (x .or. y?=w804:bool)
                n296 = Select(t=State_Type_Definitions."True Stop" ("Enum"), s=w802, f=State_Type_Definitions."Task 5 _B" ("Enum")) -> (s? t:f=w799:u16)
                n297 = Select(t=w799, s=w804, f=State_Type_Definitions."Task 5_C_Error" ("Enum")) -> (s? t:f=w803:u16)
              }
              frame "Exit" {
                n298 = for {
                  shift-right: [w826] -> w823
                  shift-left: w820 -> [w827]
                  tunnel: string[] ["STOP", "RESET ENCODERS", "RESET YAW", "ARDUINO MODE 0"] -> [w825] mode=indexing
                  n299 = Enqueue Element(queue=w827, element=w825) -> (queue out=w826:refnum<queue>)  [unwired: 2 in, 2 out]
                }
              }
            }
            n300 = Bundle By Name(cluster=w787, "yStepper desired"=w783) -> (w786:T8)
          }
          frame 25 {
            # ">>> yStepper command>>>"
            n301 = Dequeue Element(queue=w835, timeout in ms (-1)=w834, error in (no error)=w833) -> (element=w840:T7)  [unwired: 3 out]
            n302 = Equal?(x=w831, y=u8 80) -> (x = y?=w830:bool)
            n303 = case shown="\"None\", Default" w840 {
              tunnel: [w847 State_Type_Definitions."True Stop" ("Enum")] -> w838
              tunnel: [w846 w864] -> w837
              tunnel: [State_Type_Definitions."Idle" ("Enum") State_Type_Definitions."Shutdown" ("Enum")] -> w839
              tunnel: w836 -> [w842 _]
              tunnel: w832 -> [w844 _]
              tunnel: w830 -> [w841 _]
              frame "None", Default {
                n304 = case shown="False" w841 {
                  tunnel: [w852 w858] -> w846
                  tunnel: w844 -> [w850 w856]
                  frame False {
                    n305 = for {
                      tunnel: string[] ["Z STEPPER CAM HEIGHT", "READ STEPPER VALUES"] ("element") -> [w853] mode=indexing
                      shift-right: [w855] -> w852
                      shift-left: w850 -> [w854]
                      n306 = Enqueue Element(queue=w854, element=w853) -> (queue out=w855:refnum<queue>)  [unwired: 2 in, 2 out]
                    }
                  }
                  frame True {
                    n307 = for {
                      shift-right: [w860] -> w858
                      shift-left: w856 -> [w861]
                      tunnel: string[] ["CAM ACQ", ""] -> [w859] mode=indexing
                      n308 = Enqueue Element(queue=w861, element=w859) -> (queue out=w860:refnum<queue>)  [unwired: 2 in, 2 out]
                    }
                  }
                }
                n309 = Or(x=w841, y=w842) -> (x .or. y?=w843:bool)
                n310 = Select(t=State_Type_Definitions."Task 6_B" ("Enum"), s=w843, f=State_Type_Definitions."Task 6_A" ("Enum")) -> (s? t:f=w847:T6)
              }
              frame "Exit" {
                n311 = for {
                  shift-right: [w867] -> w864
                  shift-left: _ -> [w868]
                  tunnel: string[] ["STOP", "RESET ENCODERS", "RESET YAW", "ARDUINO MODE 0"] -> [w866] mode=indexing
                  n312 = Enqueue Element(queue=w868, element=w866) -> (queue out=w867:refnum<queue>)  [unwired: 2 in, 2 out]
                }
              }
            }
          }
          frame 26 {
            # ">>> yStepper command>>>"
            n313 = Dequeue Element(queue=w878, timeout in ms (-1)=w876, error in (no error)=w877) -> (element=w875:T7)  [unwired: 3 out]
            n314 = case shown="\"None\", Default" w875 {
              tunnel: [w885 State_Type_Definitions."True Stop" ("Enum")] -> w871
              tunnel: [w884 w903] -> w879
              tunnel: [State_Type_Definitions."Idle" ("Enum") State_Type_Definitions."Shutdown" ("Enum")] -> w872
              tunnel: w874 -> [w880 _]
              tunnel: w873 -> [w882 _]
              tunnel: w870 -> [w881 w900]
              frame "None", Default {
                # ">> Manual override >>"
                n315 = case shown="False" w882 {
                  tunnel: [w890 w896] -> w884
                  tunnel: w881 -> [w889 w894]
                  frame False {
                    n316 = for {
                      shift-right: [w893] -> w890
                      shift-left: w889 -> [w892]
                      tunnel: string[] ["CAM ACQ", "PROCESS IMAGE", "OPEN CLAW"] -> [w891] mode=indexing
                      n317 = Enqueue Element(queue=w892, element=w891) -> (queue out=w893:refnum<queue>)  [unwired: 2 in, 2 out]
                    }
                  }
                  frame True {
                    n318 = for {
                      shift-right: [w898] -> w896
                      shift-left: w894 -> [w899]
                      tunnel: string[] ["CAM ACQ", "PROCESS IMAGE", "CLOSE CLAW"] -> [w897] mode=indexing
                      n319 = Enqueue Element(queue=w899, element=w897) -> (queue out=w898:refnum<queue>)  [unwired: 2 in, 2 out]
                    }
                  }
                }
                n320 = Select(t=State_Type_Definitions."True Stop" ("Enum"), s=w880, f=State_Type_Definitions."Task 6_B" ("Enum")) -> (s? t:f=w885:T6)
              }
              frame "Exit" {
                # ">> State after true stop >>"
                # ">> Goes to true stop >>"
                n321 = for {
                  shift-right: [w906] -> w903
                  shift-left: w900 -> [w907]
                  tunnel: string[] ["STOP", "RESET ENCODERS", "RESET YAW", ""] -> [w905] mode=indexing
                  n322 = Enqueue Element(queue=w907, element=w905) -> (queue out=w906:refnum<queue>)  [unwired: 2 in, 2 out]
                }
              }
            }
          }
        }
      }
    }
  }
  n323 = call <vilib>:"DIO Close.vi"("error in (no error)"=w24, "DIO Info In"=w27) -> ()  [unwired: 9 in, 1 out]
  n324 = call <vilib>:"DIO Close.vi"("error in (no error)"=w34, "DIO Info In"=w36) -> ()  [unwired: 9 in, 1 out]
  n325 = call <vilib>:"NavX Close.vi"("error in (no error)"=w5, "NavX Info In"=w4) -> ()  [unwired: 9 in, 1 out]
  n326 = call <vilib>:"DIO Close.vi"("error in (no error)"=w29, "DIO Info In"=w31) -> ()  [unwired: 9 in, 1 out]
  n327 = call <vilib>:"DIO Close.vi"("error in (no error)"=w12, "DIO Info In"=w13) -> ()  [unwired: 9 in, 1 out]
  n328 = call <vilib>:"DIO Close.vi"("error in (no error)"=w7, "DIO Info In"=w8) -> ()  [unwired: 9 in, 1 out]
  n329 = while {
    stop <- w1330 stop-if-true
    n330 = call <vilib>:"RT Get CPU Loads.vi"() -> ("CPU loads"=→"CPU loads":T5[])  [unwired: 10 in, 1 out]
    n331 = Wait (ms)(milliseconds to wait=u32 100) -> ()  [unwired: 1 out]
    n332 = call "FGV Bool.vi"("Init/Read/Write State"=States_for_Action_Engine."Read") -> ("Output node"=w1330:bool)  [unwired: 2 in, 1 out]
  }
  n333 = Merge Errors "Merge Errors"(w64, w63) -> (w46:errorcluster)
  n334 = Merge Errors(w50, w46) -> (w45:errorcluster)
  n335 = Destroy User Event(user event=w67, error in=w45) -> ()  [unwired: 1 out]
  n336 = Destroy User Event(user event=w68, error in=w45) -> ()  [unwired: 1 out]
  n337 = Unregister For Events(event registration refnum=w59, error in=w45) -> ()  [unwired: 1 out]
  n338 = Release Queue(queue=w41, error in (no error)=w45) -> (error out=w23:errorcluster)  [unwired: 1 in, 2 out]
  n339 = Release Queue(queue=w58, error in (no error)=w45) -> ()  [unwired: 1 in, 3 out]
  n340 = call <vilib>:"Simple Error Handler.vi"("error in (no error)"=w23) -> ("error out"=w22:errorcluster)  [unwired: 4 in, 4 out]
  n341 = call <vilib>:"Reset myRIO.vi"("error in (no error)"=w22) -> ("error out"=→"error out":errorcluster)  [unwired: 10 in]
